vi "FlexRay_Demo.vi"(11 "Receiver":string="FlexRay_Demo") -> ()   [LabVIEW 2014]
uses:
  <vilib>/Utility/miscctls.llb/LVPointTypeDef.ctl
  TSMaster_API/FlexRay_Function/Typedef/FlexRay_Data.ctl
  TSMaster_API/FlexRay_Function/Typedef/TLibFLexRay.ctl
  TSMaster_API/FlexRay_Function/Typedef/FlexRay_Config.ctl
  TSMaster_API/DataBase/Typedef/FlexRay/TFlexRaySignal.ctl
  TSMaster_API/DataBase/Typedef/LIN/TLINSignal.ctl
  TSMaster_API/DataBase/Typedef/CAN/TCANSignal.ctl
  TSMaster_API/DataBase/Typedef/TDBSignalProperties.ctl
  TSMaster_API/DataBase/Typedef/TDBFrameProperties.ctl
  TSMaster_API/DataBase/Typedef/TDBECUProperties.ctl
  TSMaster_API/DataBase/Typedef/TDBProperties.ctl
  <vilib>/regexp/Match Regular Expression.xnode
  TSMaster_API/DataBase/Typedef/DataBase_array.ctl
  TSMaster_API/DataBase/Typedef/DataBase_array_index.ctl
panel:
  out "DataBase_array":T1
  in  "CH_Mapping":bool
  in  "TS_Mapping":bool
  in  "Diagram shown":bool
  out "FlexRay_Data":T9={"Communication message"={"Sender"="", "receiver"="", "message"="", "data"=variant}, "error in"={"status"=FALSE, "code"=0, "source"=""}, "Data"={"FR_Frame_Buffer"=[], "Config"={"DLL_PATH"=path "", "Project_PATH"=path "", "BLF_Log_PATH"=path "", "Read message type"=1, "Channel"=0, "REC_Channel"=0, "ChannelMask"=0, "ActualPayloadLength"=0, "CycleNumber"=0, "SlotId"=0, "Send_Array"=[1, 2, 3, 4, 5, 6, 7, 8, 9, 10, 11]}, "AsynCall?"=FALSE, "XML_Data"={"XML Path"=path "", "XML loading channel"=0}, "DataBase_array"=refnum}} {"Data"."XML_Data"."XML loading channel" items=["CHN1", "CHN2", "CHN3", "CHN4", "CHN5", "CHN6", "CHN7", "CHN8", "CHN9", "CHN10", "CHN11", "CHN12", "CHN13", "CHN14", "CHN15", "CHN16", "CHN17", "CHN18", "CHN19", "CHN20", "CHN21", "CHN22", "CHN23", "CHN24", "CHN25", "CHN26", "CHN27", "CHN28", "CHN29", "CHN30", "CHN31", "CHN32"]; "Data"."Config"."Send_Array" format="%.0x"; "Data"."Config"."ChannelMask" items=["reserved", "A", "B", "AB"]; "Data"."Config"."REC_Channel" items=["CHN1", "CHN2", "CHN3", "CHN4", "CHN5", "CHN6", "CHN7", "CHN8", "CHN9", "CHN10", "CHN11", "CHN12", "CHN13", "CHN14", "CHN15", "CHN16", "CHN17", "CHN18", "CHN19", "CHN20", "CHN21", "CHN22", "CHN23", "CHN24", "CHN25", "CHN26", "CHN27", "CHN28", "CHN29", "CHN30", "CHN31", "CHN32"]; "Data"."Config"."Channel" items=["CHN1", "CHN2", "CHN3", "CHN4", "CHN5", "CHN6", "CHN7", "CHN8", "CHN9", "CHN10", "CHN11", "CHN12", "CHN13", "CHN14", "CHN15", "CHN16", "CHN17", "CHN18", "CHN19", "CHN20", "CHN21", "CHN22", "CHN23", "CHN24", "CHN25", "CHN26", "CHN27", "CHN28", "CHN29", "CHN30", "CHN31", "CHN32"]; "Data"."Config"."Read message type" items=["Only read received messages", "Receive&send messages"]}
  in  "Stop Log":bool
  in  "Start Log":bool
  in  "Config":bool
  in  "Connect":bool
  in  "Disconnect":bool
  out "Connect ?":bool
  in  "Tab Control":enum32{"Setting", "FlexRay", "XML_load"}(tab)
  in  "BLF_Log_PATH":path
  in  "Project_PATH":path
  in  "DLL_PATH":path
  in  "Import":bool
  in  "Export":bool
  in  "Signals":string[][](array[string])
  in  "Messages":string(combo)
  in  "Fold Data":bool
  in  "Transmit":bool
  in  "Send_Array":u8[](array[numeric])=[1, 2, 3, 4, 5, 6, 7, 8, 9, 10, 11] format="%.0x"
  in  "SlotId":u16
  in  "CycleNumber":u8 caption="Base+Rep"
  in  "ActualPayloadLength":u8 caption="Length"
  in  "DIS_REC":bool
  in  "Clear":bool
  in  "Pause":bool
  in  "REC_Channel":i32(ring) items=["CHN1", "CHN2", "CHN3", "CHN4", "CHN5", "CHN6", "CHN7", "CHN8", "CHN9", "CHN10", "CHN11", "CHN12", "CHN13", "CHN14", "CHN15", "CHN16", "CHN17", "CHN18", "CHN19", "CHN20", "CHN21", "CHN22", "CHN23", "CHN24", "CHN25", "CHN26", "CHN27", "CHN28", "CHN29", "CHN30", "CHN31", "CHN32"]
  in  "Channel":i32(ring) caption="REC_Channel" items=["CHN1", "CHN2", "CHN3", "CHN4", "CHN5", "CHN6", "CHN7", "CHN8", "CHN9", "CHN10", "CHN11", "CHN12", "CHN13", "CHN14", "CHN15", "CHN16", "CHN17", "CHN18", "CHN19", "CHN20", "CHN21", "CHN22", "CHN23", "CHN24", "CHN25", "CHN26", "CHN27", "CHN28", "CHN29", "CHN30", "CHN31", "CHN32"]
  out "Receive Status":bool
  in  "Read message type":u16(ring)=1 items=["Only read received messages", "Receive&send messages"]
  in  "Receive_Data":i32(listbox)=-1 caption="Data"
  in  "ChannelMask":u16(ring) items=["reserved", "A", "B", "AB"]
  out "Laod XML Successful?":bool caption="Laod BDC Successful?"
  in  "Unload":bool
  in  "Load_XML":bool
  in  "XML loading channel":i32(ring) items=["CHN1", "CHN2", "CHN3", "CHN4", "CHN5", "CHN6", "CHN7", "CHN8", "CHN9", "CHN10", "CHN11", "CHN12", "CHN13", "CHN14", "CHN15", "CHN16", "CHN17", "CHN18", "CHN19", "CHN20", "CHN21", "CHN22", "CHN23", "CHN24", "CHN25", "CHN26", "CHN27", "CHN28", "CHN29", "CHN30", "CHN31", "CHN32"]
  in  "XML Path":path
  in  "XML Tab":enum32{"Message", "Signal"}(tab) caption="Tab Control 2"
  in  "Message Table":string[][](table)=[["Name", ""], ["ChannelMask", ""], ["BaseCycle", ""], ["CycleRepetition", ""], ["SlotId", ""], ["DLC", ""], ["", ""], ["", ""]]
  in  "Signal Table":string[][](table)
  in  "Tree control":string(tree)
  in  "Creat error":bool
  in  "log":i32(listbox)
  in  "Quit":bool
  # "FlexRay Demo"
  # "Please click the 'Config' button first,Don't click \"Connect\""
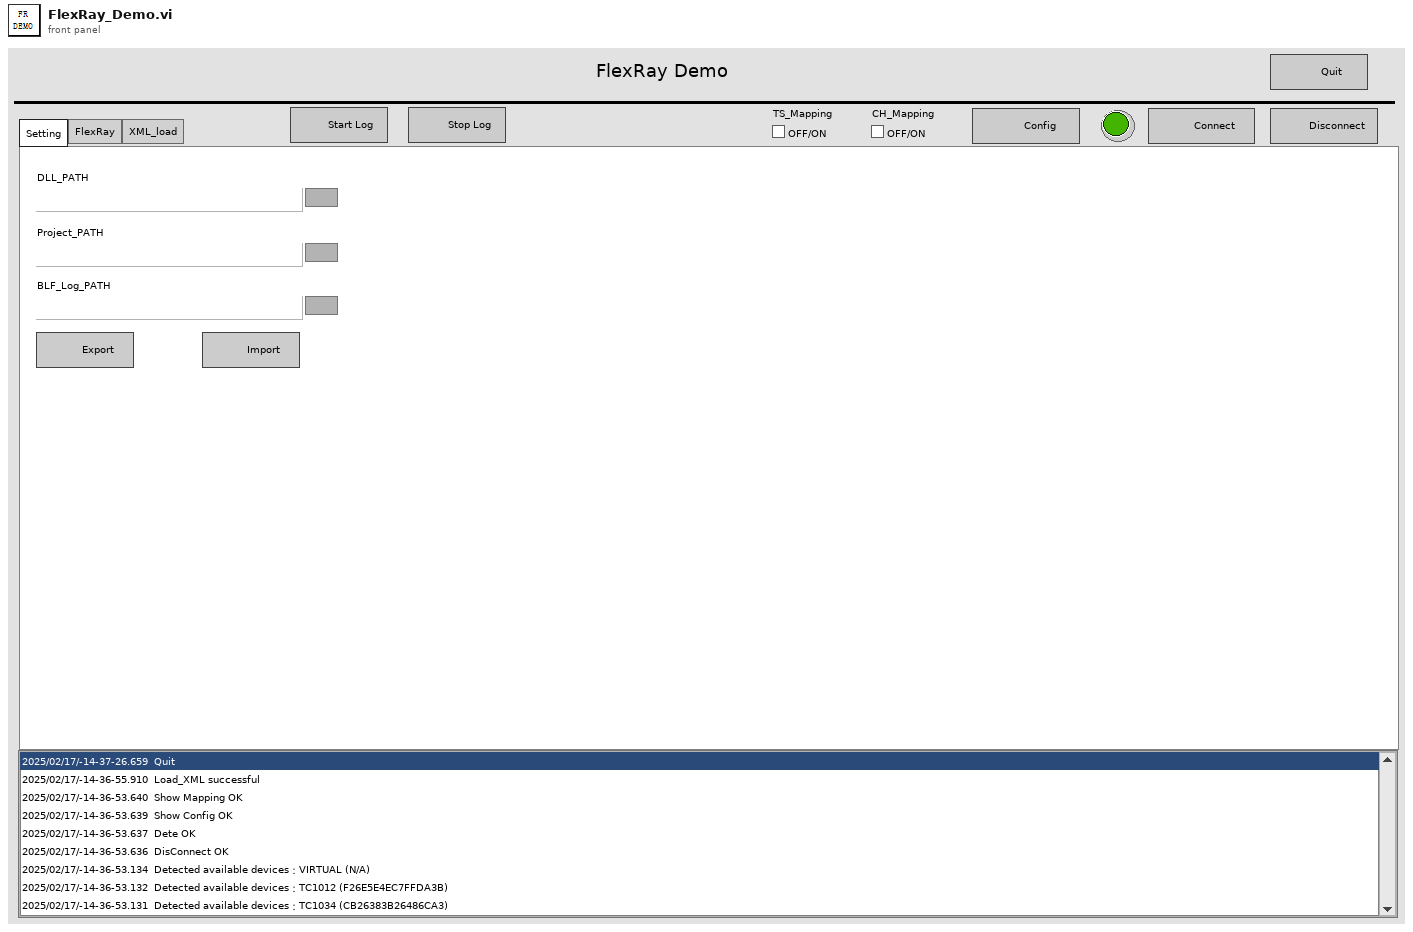
[diagram p1: front panel]
types:
  T1 = typedef "DataBase_array.ctl" = cluster{"db_properties":T2, "ECU_array":cluster{"TDBECUProperties":T3, "TX_Frame_array":cluster{"Frame_Properties":T4, "signal_array":T5[]}[], "RX_Frame_array":cluster{"Frame_Properties":T4, "signal_array":T5[]}[]}[]}[]
  T2 = typedef "TDBProperties.ctl" = cluster{"FDBIndex":i32, "FSignalCount":i32, "FFrameCount":i32, "FECUCount":i32, "FSupportedChannelMask":u64, "FName":cluster{"数值":u64, "数值 2":u64, "数值 3":u64, "数值 4":u64, "数值 5":u64, "数值 6":u64, "数值 7":u64, "数值 8":u64, "数值 9":u64, "数值 10":u64, "数值 11":u64, "数值 12":u64, "数值 13":u64, "数值 14":u64, "数值 15":u64, "数值 16":u64, "数值 17":u64, "数值 18":u64, "数值 19":u64, "数值 20":u64, "数值 21":u64, "数值 22":u64, "数值 23":u64, "数值 24":u64, "数值 25":u64, "数值 26":u64, "数值 27":u64, "数值 28":u64, "数值 29":u64, "数值 30":u64, "数值 31":u64, "数值 32":u64, "数值 33":u64, "数值 34":u64, "数值 35":u64, "数值 36":u64, "数值 37":u64, "数值 38":u64, "数值 39":u64, "数值 40":u64, "数值 41":u64, "数值 42":u64, "数值 43":u64, "数值 44":u64, "数值 45":u64, "数值 46":u64, "数值 47":u64, "数值 48":u64, "数值 49":u64, "数值 50":u64, "数值 51":u64, "数值 52":u64, "数值 53":u64, "数值 54":u64, "数值 55":u64, "数值 56":u64, "数值 57":u64, "数值 58":u64, "数值 59":u64, "数值 60":u64, "数值 61":u64, "数值 62":u64, "数值 63":u64, "数值 64":u64}, "FComment":cluster{"数值":u64, "数值 2":u64, "数值 3":u64, "数值 4":u64, "数值 5":u64, "数值 6":u64, "数值 7":u64, "数值 8":u64, "数值 9":u64, "数值 10":u64, "数值 11":u64, "数值 12":u64, "数值 13":u64, "数值 14":u64, "数值 15":u64, "数值 16":u64, "数值 17":u64, "数值 18":u64, "数值 19":u64, "数值 20":u64, "数值 21":u64, "数值 22":u64, "数值 23":u64, "数值 24":u64, "数值 25":u64, "数值 26":u64, "数值 27":u64, "数值 28":u64, "数值 29":u64, "数值 30":u64, "数值 31":u64, "数值 32":u64, "数值 33":u64, "数值 34":u64, "数值 35":u64, "数值 36":u64, "数值 37":u64, "数值 38":u64, "数值 39":u64, "数值 40":u64, "数值 41":u64, "数值 42":u64, "数值 43":u64, "数值 44":u64, "数值 45":u64, "数值 46":u64, "数值 47":u64, "数值 48":u64, "数值 49":u64, "数值 50":u64, "数值 51":u64, "数值 52":u64, "数值 53":u64, "数值 54":u64, "数值 55":u64, "数值 56":u64, "数值 57":u64, "数值 58":u64, "数值 59":u64, "数值 60":u64, "数值 61":u64, "数值 62":u64, "数值 63":u64, "数值 64":u64}, "FFlags":u32, "FDBId":u32}
  T3 = typedef "TDBECUProperties.ctl" = cluster{"FDBIndex":i32, "FECUIndex":i32, "FTxFrameCount":i32, "FRxFrameCount":i32, "FName":cluster{"数值":u64, "数值 2":u64, "数值 3":u64, "数值 4":u64, "数值 5":u64, "数值 6":u64, "数值 7":u64, "数值 8":u64, "数值 9":u64, "数值 10":u64, "数值 11":u64, "数值 12":u64, "数值 13":u64, "数值 14":u64, "数值 15":u64, "数值 16":u64, "数值 17":u64, "数值 18":u64, "数值 19":u64, "数值 20":u64, "数值 21":u64, "数值 22":u64, "数值 23":u64, "数值 24":u64, "数值 25":u64, "数值 26":u64, "数值 27":u64, "数值 28":u64, "数值 29":u64, "数值 30":u64, "数值 31":u64, "数值 32":u64, "数值 33":u64, "数值 34":u64, "数值 35":u64, "数值 36":u64, "数值 37":u64, "数值 38":u64, "数值 39":u64, "数值 40":u64, "数值 41":u64, "数值 42":u64, "数值 43":u64, "数值 44":u64, "数值 45":u64, "数值 46":u64, "数值 47":u64, "数值 48":u64, "数值 49":u64, "数值 50":u64, "数值 51":u64, "数值 52":u64, "数值 53":u64, "数值 54":u64, "数值 55":u64, "数值 56":u64, "数值 57":u64, "数值 58":u64, "数值 59":u64, "数值 60":u64, "数值 61":u64, "数值 62":u64, "数值 63":u64, "数值 64":u64}, "FComment":cluster{"数值":u64, "数值 2":u64, "数值 3":u64, "数值 4":u64, "数值 5":u64, "数值 6":u64, "数值 7":u64, "数值 8":u64, "数值 9":u64, "数值 10":u64, "数值 11":u64, "数值 12":u64, "数值 13":u64, "数值 14":u64, "数值 15":u64, "数值 16":u64, "数值 17":u64, "数值 18":u64, "数值 19":u64, "数值 20":u64, "数值 21":u64, "数值 22":u64, "数值 23":u64, "数值 24":u64, "数值 25":u64, "数值 26":u64, "数值 27":u64, "数值 28":u64, "数值 29":u64, "数值 30":u64, "数值 31":u64, "数值 32":u64, "数值 33":u64, "数值 34":u64, "数值 35":u64, "数值 36":u64, "数值 37":u64, "数值 38":u64, "数值 39":u64, "数值 40":u64, "数值 41":u64, "数值 42":u64, "数值 43":u64, "数值 44":u64, "数值 45":u64, "数值 46":u64, "数值 47":u64, "数值 48":u64, "数值 49":u64, "数值 50":u64, "数值 51":u64, "数值 52":u64, "数值 53":u64, "数值 54":u64, "数值 55":u64, "数值 56":u64, "数值 57":u64, "数值 58":u64, "数值 59":u64, "数值 60":u64, "数值 61":u64, "数值 62":u64, "数值 63":u64, "数值 64":u64}}
  T4 = typedef "TDBFrameProperties.ctl" = cluster{"FDBIndex":i32, "FECUIndex":i32, "FFrameIndex":i32, "FIsTx":u8, "FReserved1":u8, "FCycleTimeMs":u16, "TSignalType":i32, "FCANIsDataFrame":u8, "FCANIsStdFrame":u8, "FCANIsEdl":u8, "FCANIsBrs":u8, "FCANIdentifier":i32, "FCANDLC":i32, "FCANDataBytes":i32, "FLINIdentifier":i32, "FLINDLC":i32, "FFRChannelMask":u8, "FFRBaseCycle":u8, "FFRCycleRepetition":u8, "FFRIsStartupFrame":u8, "FFRSlotId":u16, "FFRDLC":u16, "FFRCycleMask":u64, "FSignalCount":i32, "FName":cluster{"数值":u64, "数值 2":u64, "数值 3":u64, "数值 4":u64, "数值 5":u64, "数值 6":u64, "数值 7":u64, "数值 8":u64, "数值 9":u64, "数值 10":u64, "数值 11":u64, "数值 12":u64, "数值 13":u64, "数值 14":u64, "数值 15":u64, "数值 16":u64, "数值 17":u64, "数值 18":u64, "数值 19":u64, "数值 20":u64, "数值 21":u64, "数值 22":u64, "数值 23":u64, "数值 24":u64, "数值 25":u64, "数值 26":u64, "数值 27":u64, "数值 28":u64, "数值 29":u64, "数值 30":u64, "数值 31":u64, "数值 32":u64, "数值 33":u64, "数值 34":u64, "数值 35":u64, "数值 36":u64, "数值 37":u64, "数值 38":u64, "数值 39":u64, "数值 40":u64, "数值 41":u64, "数值 42":u64, "数值 43":u64, "数值 44":u64, "数值 45":u64, "数值 46":u64, "数值 47":u64, "数值 48":u64, "数值 49":u64, "数值 50":u64, "数值 51":u64, "数值 52":u64, "数值 53":u64, "数值 54":u64, "数值 55":u64, "数值 56":u64, "数值 57":u64, "数值 58":u64, "数值 59":u64, "数值 60":u64, "数值 61":u64, "数值 62":u64, "数值 63":u64, "数值 64":u64}, "FComment":cluster{"数值":u64, "数值 2":u64, "数值 3":u64, "数值 4":u64, "数值 5":u64, "数值 6":u64, "数值 7":u64, "数值 8":u64, "数值 9":u64, "数值 10":u64, "数值 11":u64, "数值 12":u64, "数值 13":u64, "数值 14":u64, "数值 15":u64, "数值 16":u64, "数值 17":u64, "数值 18":u64, "数值 19":u64, "数值 20":u64, "数值 21":u64, "数值 22":u64, "数值 23":u64, "数值 24":u64, "数值 25":u64, "数值 26":u64, "数值 27":u64, "数值 28":u64, "数值 29":u64, "数值 30":u64, "数值 31":u64, "数值 32":u64, "数值 33":u64, "数值 34":u64, "数值 35":u64, "数值 36":u64, "数值 37":u64, "数值 38":u64, "数值 39":u64, "数值 40":u64, "数值 41":u64, "数值 42":u64, "数值 43":u64, "数值 44":u64, "数值 45":u64, "数值 46":u64, "数值 47":u64, "数值 48":u64, "数值 49":u64, "数值 50":u64, "数值 51":u64, "数值 52":u64, "数值 53":u64, "数值 54":u64, "数值 55":u64, "数值 56":u64, "数值 57":u64, "数值 58":u64, "数值 59":u64, "数值 60":u64, "数值 61":u64, "数值 62":u64, "数值 63":u64, "数值 64":u64}}
  T5 = typedef "TDBSignalProperties.ctl" = cluster{"FDBIndex":i32, "FECUIndex":i32, "FFrameIndex":i32, "FSignalIndex":i32, "FIsTx":u8, "FReserved1":u8, "FReserved2":u8, "FReserved3":u8, "TSignalType":i32, "TCANSignal":T6, "TLINSignal":T7, "TFlexRaySignal":T8, "FParentFrameId":i32, "FInitValue":dbl, "FName":cluster{"数值":u64, "数值 2":u64, "数值 3":u64, "数值 4":u64, "数值 5":u64, "数值 6":u64, "数值 7":u64, "数值 8":u64, "数值 9":u64, "数值 10":u64, "数值 11":u64, "数值 12":u64, "数值 13":u64, "数值 14":u64, "数值 15":u64, "数值 16":u64, "数值 17":u64, "数值 18":u64, "数值 19":u64, "数值 20":u64, "数值 21":u64, "数值 22":u64, "数值 23":u64, "数值 24":u64, "数值 25":u64, "数值 26":u64, "数值 27":u64, "数值 28":u64, "数值 29":u64, "数值 30":u64, "数值 31":u64, "数值 32":u64, "数值 33":u64, "数值 34":u64, "数值 35":u64, "数值 36":u64, "数值 37":u64, "数值 38":u64, "数值 39":u64, "数值 40":u64, "数值 41":u64, "数值 42":u64, "数值 43":u64, "数值 44":u64, "数值 45":u64, "数值 46":u64, "数值 47":u64, "数值 48":u64, "数值 49":u64, "数值 50":u64, "数值 51":u64, "数值 52":u64, "数值 53":u64, "数值 54":u64, "数值 55":u64, "数值 56":u64, "数值 57":u64, "数值 58":u64, "数值 59":u64, "数值 60":u64, "数值 61":u64, "数值 62":u64, "数值 63":u64, "数值 64":u64}, "FComment":cluster{"数值":u64, "数值 2":u64, "数值 3":u64, "数值 4":u64, "数值 5":u64, "数值 6":u64, "数值 7":u64, "数值 8":u64, "数值 9":u64, "数值 10":u64, "数值 11":u64, "数值 12":u64, "数值 13":u64, "数值 14":u64, "数值 15":u64, "数值 16":u64, "数值 17":u64, "数值 18":u64, "数值 19":u64, "数值 20":u64, "数值 21":u64, "数值 22":u64, "数值 23":u64, "数值 24":u64, "数值 25":u64, "数值 26":u64, "数值 27":u64, "数值 28":u64, "数值 29":u64, "数值 30":u64, "数值 31":u64, "数值 32":u64, "数值 33":u64, "数值 34":u64, "数值 35":u64, "数值 36":u64, "数值 37":u64, "数值 38":u64, "数值 39":u64, "数值 40":u64, "数值 41":u64, "数值 42":u64, "数值 43":u64, "数值 44":u64, "数值 45":u64, "数值 46":u64, "数值 47":u64, "数值 48":u64, "数值 49":u64, "数值 50":u64, "数值 51":u64, "数值 52":u64, "数值 53":u64, "数值 54":u64, "数值 55":u64, "数值 56":u64, "数值 57":u64, "数值 58":u64, "数值 59":u64, "数值 60":u64, "数值 61":u64, "数值 62":u64, "数值 63":u64, "数值 64":u64}}
  T6 = typedef "TCANSignal.ctl" = cluster{"FCANSgnType":u8, "FIsIntel":u8, "FStartBit":i32, "FLength":i32, "FFactor":dbl, "FOffset":dbl}
  T7 = typedef "TLINSignal.ctl" = cluster{"FLINSgnType":u8, "FIsIntel":u8, "FStartBit":i32, "FLength":i32, "FFactor":dbl, "FOffset":dbl}
  T8 = typedef "TFlexRaySignal.ctl" = cluster{"FFRSgnType":u8, "FCompuMethod":u8, "FReserved":u8, "FIsIntel":u8, "FStartBit":i32, "FUpdateBit":i32, "FLength":i32, "FFactor":dbl, "FOffset":dbl, "FActualStartBit":i32, "FActualUpdateBit":i32}
  T9 = typedef "FlexRay_Data.ctl" = cluster{"Communication message":cluster{"Sender":string, "receiver":string, "message":string, "data":variant}, "error in":errorcluster, "Data":cluster{"FR_Frame_Buffer":T10[], "Config":T11, "AsynCall?":bool, "XML_Data":cluster{"XML Path":path, "XML loading channel":i32}, "DataBase_array":T12}}
  T10 = typedef "TLibFLexRay.ctl" = cluster{"FIdxChn":u8, "FChannelMask":u8, "FDir":u8, "FPayloadLength":u8, "FActualPayloadLength":u8, "FCycleNumber":u8, "FCCType":u8, "FFrameType":u8, "FHeaderCRCA":u16, "FHeaderCRCB":u16, "FFrameStateInfo":u16, "FSlotId":u16, "FFrameFlags":u32, "FFrameCRC":u32, "FReserved1":u64, "FReserved2":u64, "FTimeUs":u64, "FData":cluster{"数值":u8, "数值 9":u8, "数值 17":u8, "数值 25":u8, "数值 33":u8, "数值 41":u8, "数值 49":u8, "数值 57":u8, "数值 65":u8, "数值 73":u8, "数值 81":u8, "数值 89":u8, "数值 97":u8, "数值 105":u8, "数值 98":u8, "数值 99":u8, "数值 2":u8, "数值 10":u8, "数值 18":u8, "数值 26":u8, "数值 34":u8, "数值 42":u8, "数值 50":u8, "数值 58":u8, "数值 66":u8, "数值 74":u8, "数值 82":u8, "数值 90":u8, "数值 100":u8, "数值 106":u8, "数值 101":u8, "数值 102":u8, "数值 3":u8, "数值 11":u8, "数值 19":u8, "数值 27":u8, "数值 35":u8, "数值 43":u8, "数值 51":u8, "数值 59":u8, "数值 67":u8, "数值 75":u8, "数值 83":u8, "数值 91":u8, "数值 103":u8, "数值 107":u8, "数值 104":u8, "数值 108":u8, "数值 4":u8, "数值 12":u8, "数值 20":u8, "数值 28":u8, "数值 36":u8, "数值 44":u8, "数值 52":u8, "数值 60":u8, "数值 68":u8, "数值 76":u8, "数值 84":u8, "数值 92":u8, "数值 109":u8, "数值 110":u8, "数值 111":u8, "数值 112":u8, "数值 5":u8, "数值 13":u8, "数值 21":u8, "数值 29":u8, "数值 37":u8, "数值 45":u8, "数值 53":u8, "数值 61":u8, "数值 69":u8, "数值 77":u8, "数值 85":u8, "数值 93":u8, "数值 113":u8, "数值 114":u8, "数值 115":u8, "数值 116":u8, "数值 6":u8, "数值 14":u8, "数值 22":u8, "数值 30":u8, "数值 38":u8, "数值 46":u8, "数值 54":u8, "数值 62":u8, "数值 70":u8, "数值 78":u8, "数值 86":u8, "数值 94":u8, "数值 117":u8, "数值 118":u8, "数值 119":u8, "数值 120":u8, "数值 7":u8, "数值 15":u8, "数值 23":u8, "数值 31":u8, "数值 39":u8, "数值 47":u8, "数值 55":u8, "数值 63":u8, "数值 71":u8, "数值 79":u8, "数值 87":u8, "数值 95":u8, "数值 121":u8, "数值 122":u8, "数值 123":u8, "数值 124":u8, "数值 8":u8, "数值 16":u8, "数值 24":u8, "数值 32":u8, "数值 40":u8, "数值 48":u8, "数值 56":u8, "数值 64":u8, "数值 72":u8, "数值 80":u8, "数值 88":u8, "数值 96":u8, "数值 125":u8, "数值 126":u8, "数值 127":u8, "数值 128":u8, "数值 129":u8, "数值 130":u8, "数值 131":u8, "数值 132":u8, "数值 133":u8, "数值 134":u8, "数值 135":u8, "数值 136":u8, "数值 137":u8, "数值 138":u8, "数值 139":u8, "数值 140":u8, "数值 141":u8, "数值 142":u8, "数值 143":u8, "数值 144":u8, "数值 145":u8, "数值 146":u8, "数值 147":u8, "数值 148":u8, "数值 149":u8, "数值 150":u8, "数值 151":u8, "数值 152":u8, "数值 153":u8, "数值 154":u8, "数值 155":u8, "数值 156":u8, "数值 157":u8, "数值 158":u8, "数值 159":u8, "数值 160":u8, "数值 161":u8, "数值 162":u8, "数值 163":u8, "数值 164":u8, "数值 165":u8, "数值 166":u8, "数值 167":u8, "数值 168":u8, "数值 169":u8, "数值 170":u8, "数值 171":u8, "数值 172":u8, "数值 173":u8, "数值 174":u8, "数值 175":u8, "数值 176":u8, "数值 177":u8, "数值 178":u8, "数值 179":u8, "数值 180":u8, "数值 181":u8, "数值 182":u8, "数值 183":u8, "数值 184":u8, "数值 185":u8, "数值 186":u8, "数值 187":u8, "数值 188":u8, "数值 189":u8, "数值 190":u8, "数值 191":u8, "数值 192":u8, "数值 193":u8, "数值 194":u8, "数值 195":u8, "数值 196":u8, "数值 197":u8, "数值 198":u8, "数值 199":u8, "数值 200":u8, "数值 201":u8, "数值 202":u8, "数值 203":u8, "数值 204":u8, "数值 205":u8, "数值 206":u8, "数值 207":u8, "数值 208":u8, "数值 209":u8, "数值 210":u8, "数值 211":u8, "数值 212":u8, "数值 213":u8, "数值 214":u8, "数值 215":u8, "数值 216":u8, "数值 217":u8, "数值 218":u8, "数值 219":u8, "数值 220":u8, "数值 221":u8, "数值 222":u8, "数值 223":u8, "数值 224":u8, "数值 225":u8, "数值 226":u8, "数值 227":u8, "数值 228":u8, "数值 229":u8, "数值 230":u8, "数值 231":u8, "数值 232":u8, "数值 233":u8, "数值 234":u8, "数值 235":u8, "数值 236":u8, "数值 237":u8, "数值 238":u8, "数值 239":u8, "数值 241":u8, "数值 242":u8, "数值 243":u8, "数值 244":u8, "数值 245":u8, "数值 246":u8, "数值 247":u8, "数值 248":u8, "数值 249":u8, "数值 250":u8, "数值 251":u8, "数值 252":u8, "数值 253":u8, "数值 254":u8, "数值 255":u8}}
  T11 = typedef "FlexRay_Config.ctl" = cluster{"DLL_PATH":path, "Project_PATH":path, "BLF_Log_PATH":path, "Read message type":u16, "Channel":i32, "REC_Channel":i32, "ChannelMask":u16, "ActualPayloadLength":u8, "CycleNumber":u8, "SlotId":u16, "Send_Array":u8[]}
  T12 = typedef "DataBase_array_index.ctl" = refnum<vi>
  T13 = typedef "LVPointTypeDef.ctl" = cluster{"Horizontal":i16, "Vertical":i16}
  T14 = enum8{"Enabled", "Disabled", "Disabled and Grayed Out"}
  T15 = cluster{"Sender":string, "receiver":string, "message":string, "data":variant}
  T16 = cluster{"FIdxChn":u8, "FChannelMask":u8, "FActualPayloadLength":u8, "FCycleNumber":u8, "FSlotId":u16, "Send_Array":u8[]}
  T17 = cluster{"Frame_Properties":T4, "signal_array":T5[]}
  T18 = cluster{"FR_Frame_Buffer":T10[], "Config":T11, "AsynCall?":bool, "XML_Data":cluster{"XML Path":path, "XML loading channel":i32}, "DataBase_array":T12}
  T19 = enum32{"invalid app kind", "Development System", "Run Time System", "Student Edition", "Embedded LabVIEW", "Evaluation", "Custom"}
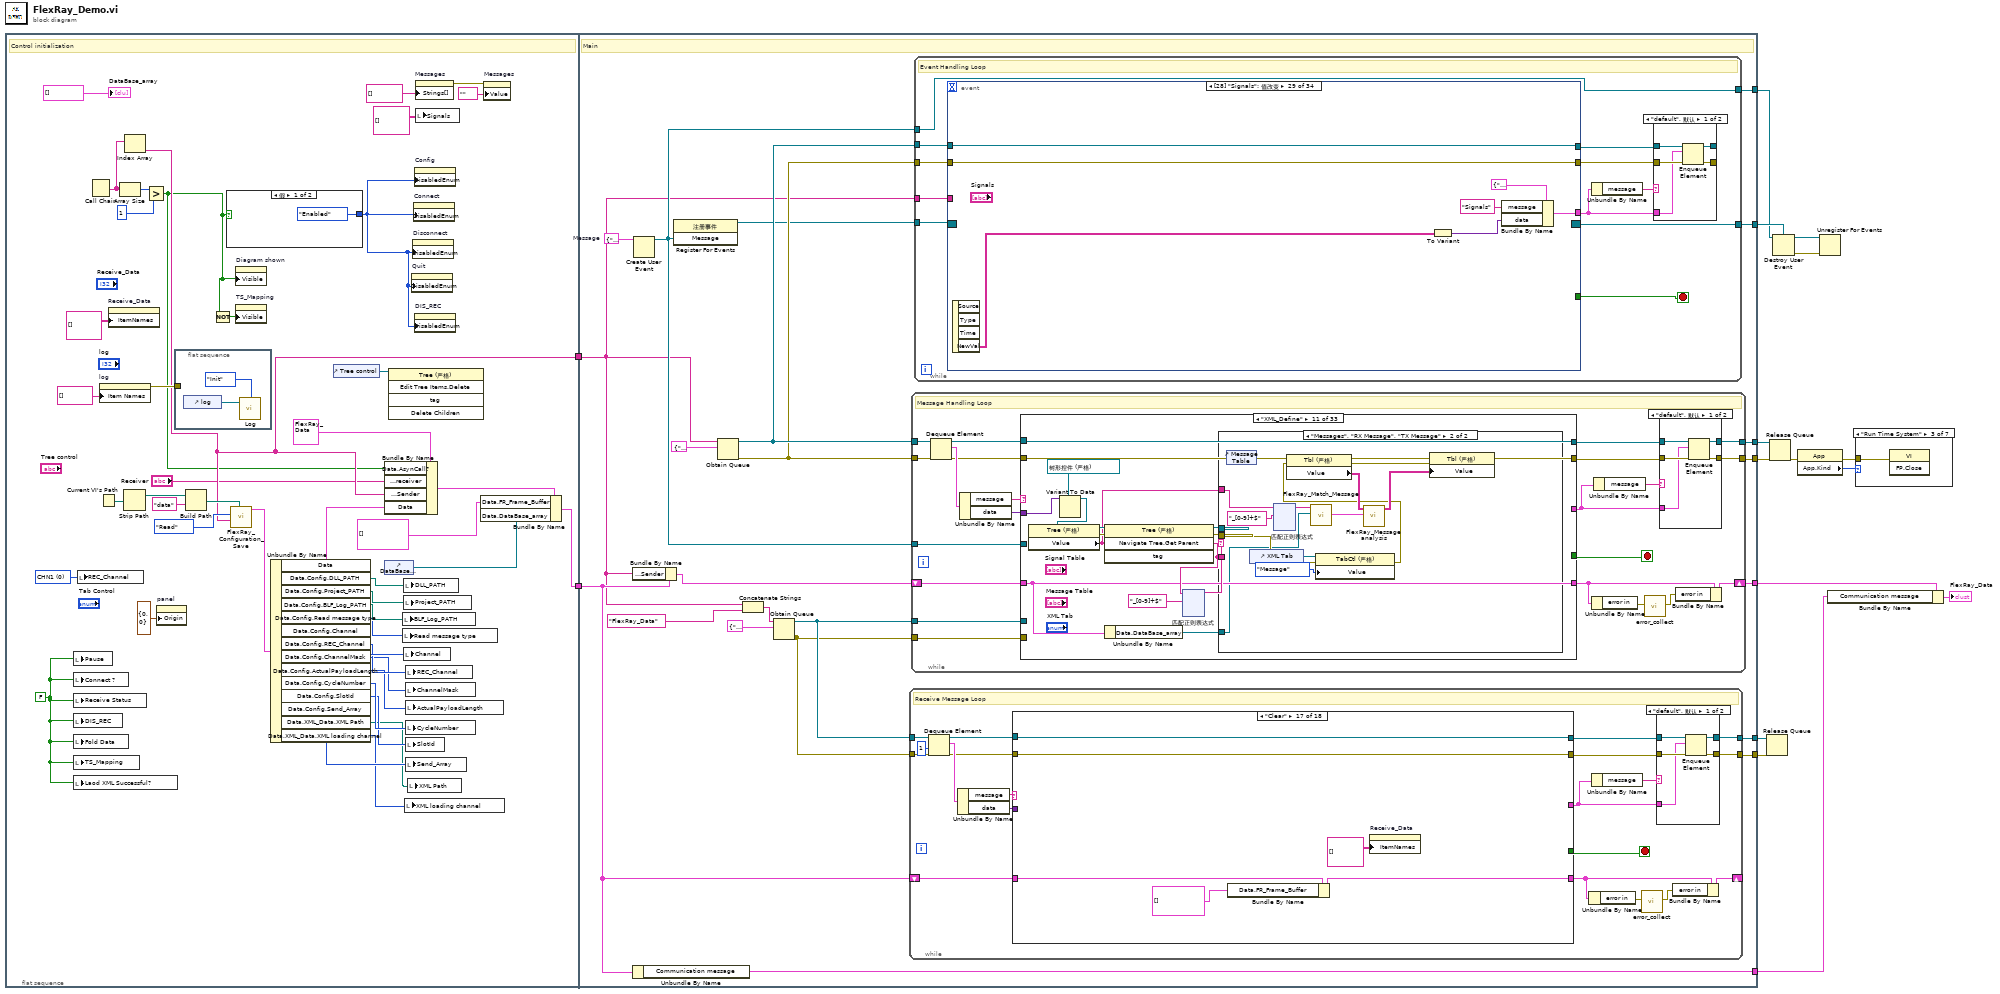
[diagram p0: block diagram]
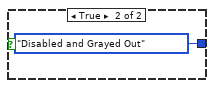
[diagram p2: hidden frame]
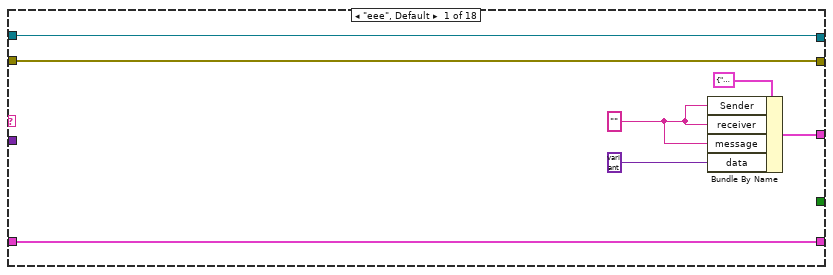
[diagram p4: hidden frame]
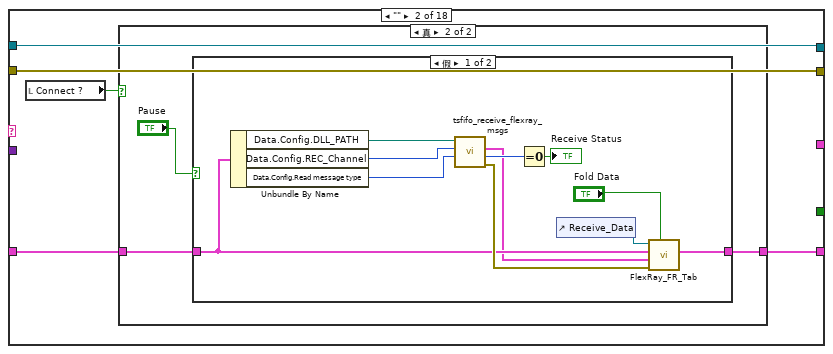
[diagram p5: hidden frame]
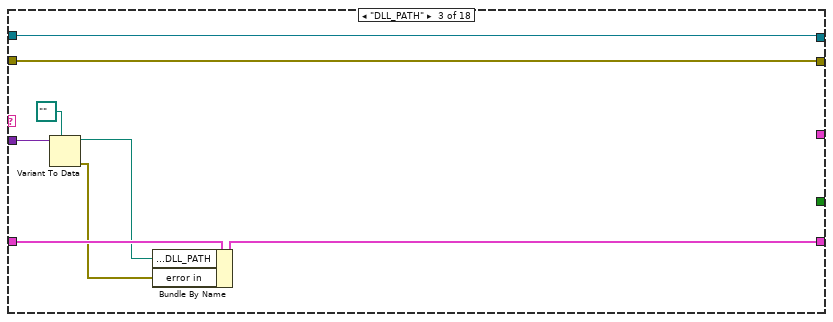
[diagram p8: hidden frame]
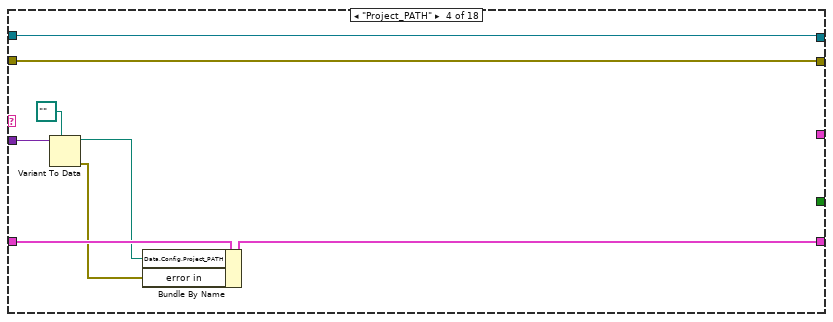
[diagram p9: hidden frame]
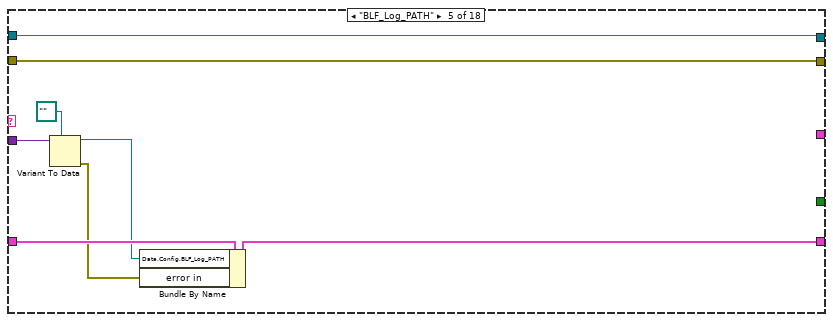
[diagram p10: hidden frame]
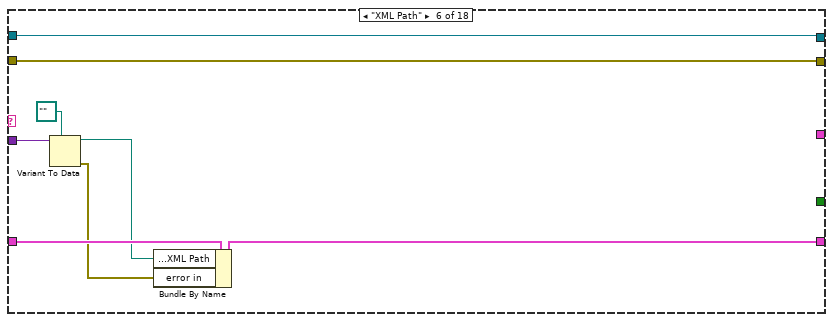
[diagram p11: hidden frame]
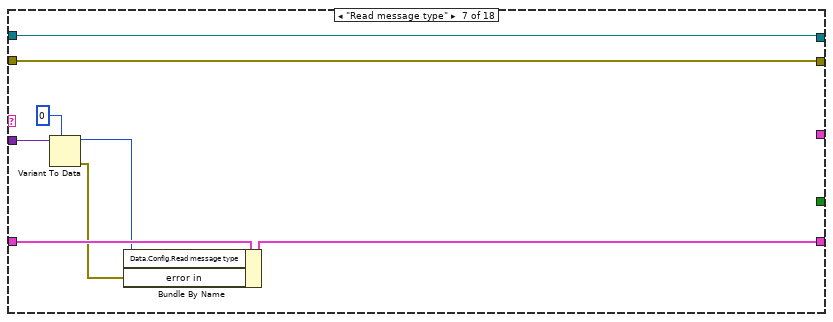
[diagram p12: hidden frame]
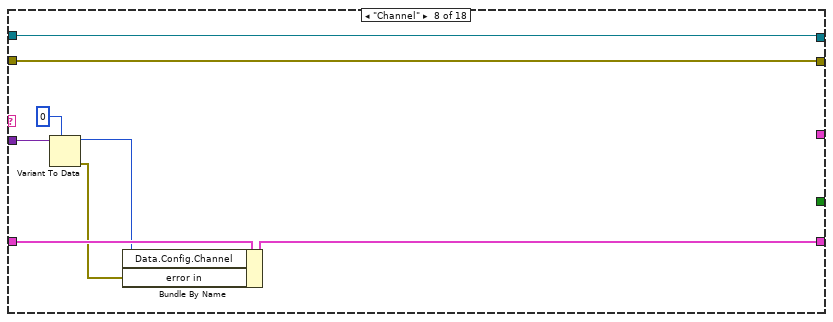
[diagram p13: hidden frame]
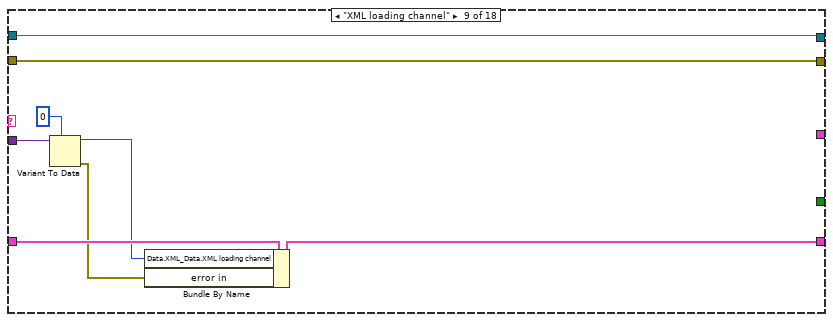
[diagram p14: hidden frame]
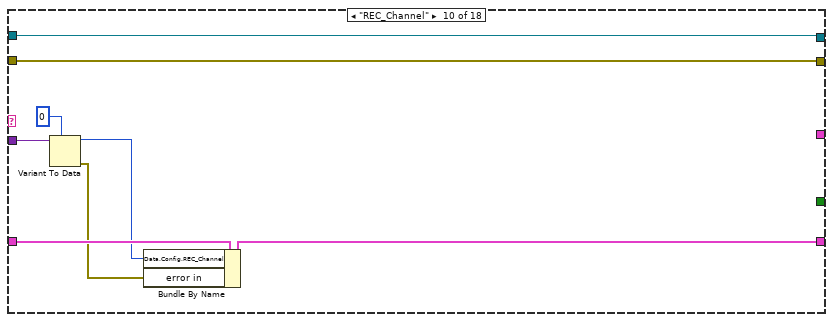
[diagram p15: hidden frame]
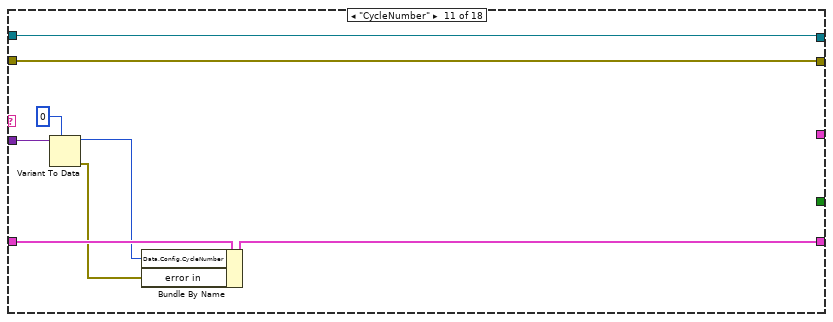
[diagram p16: hidden frame]
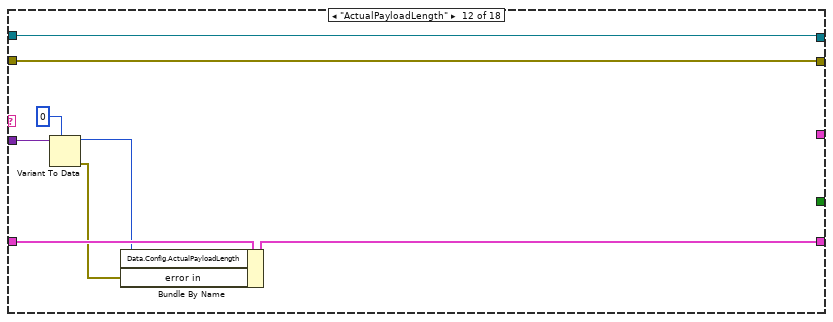
[diagram p17: hidden frame]
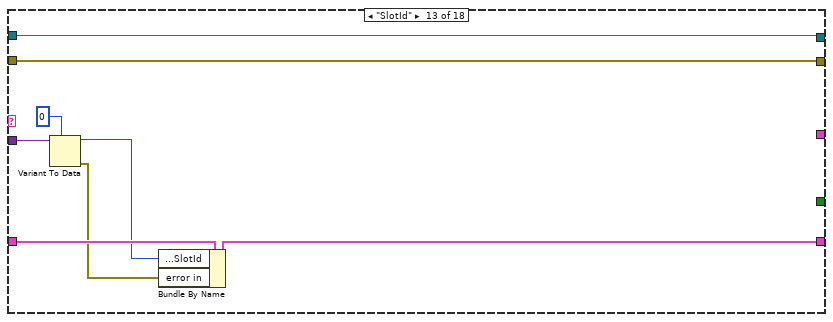
[diagram p18: hidden frame]
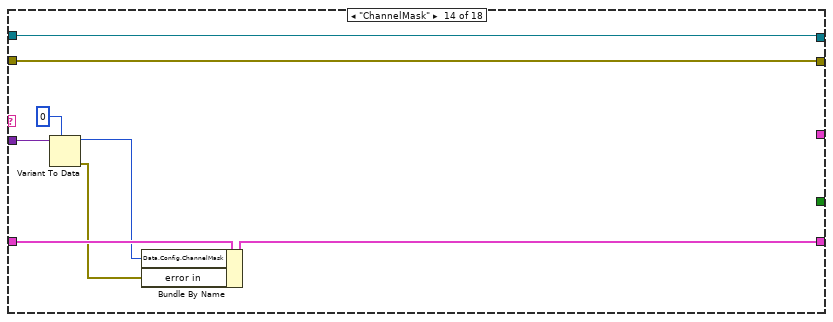
[diagram p19: hidden frame]
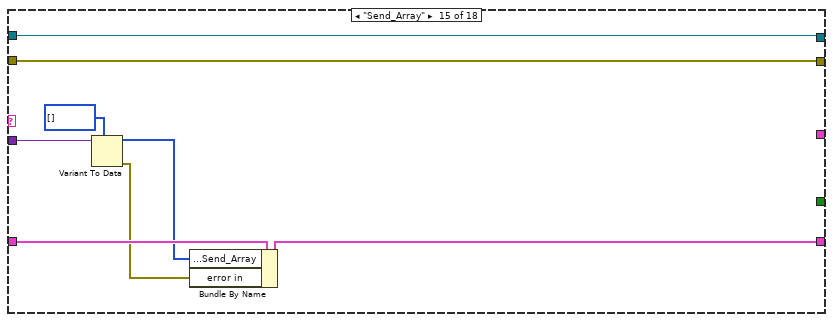
[diagram p20: hidden frame]
diagram:
  n1 = flat-sequence {
    tunnel: [w19] -> w3
    tunnel: [w33] -> w2
    tunnel: [w85] -> w15
    tunnel: [w84] -> w14
    tunnel: [w79] -> w10
    tunnel: [w77] -> w8
    tunnel: [w76] -> w7
    tunnel: [w70] -> w6
    tunnel: [w69] -> w5
    tunnel: w3 -> [w67]
    tunnel: w2 -> [w66]
    tunnel: [w68] -> w1
    frame #0 {
      w45 = 0 items=["CHN1", "CHN2", "CHN3", "CHN4", "CHN5", "CHN6", "CHN7", "CHN8", "CHN9", "CHN10", "CHN11", "CHN12", "CHN13", "CHN14", "CHN15", "CHN16", "CHN17", "CHN18", "CHN19", "CHN20", "CHN21", "CHN22", "CHN23", "CHN24", "CHN25", "CHN26", "CHN27", "CHN28", "CHN29", "CHN30", "CHN31", "CHN32"] ("REC_Channel")
      w28 = FALSE ("Connect ?")
      # "Control initialization"
      n2 = local write "Pause"(w28) -> ()
      n3 = local write "Connect ?"(w28) -> ()
      n4 = local write "Receive Status"(w28) -> ()
      n5 = local write "DIS_REC"(w28) -> ()
      n6 = local write "Fold Data"(w28) -> ()
      n7 = local write "TS_Mapping"(w28) -> ()
      n8 = local write "Laod XML Successful?"(w28) -> ()
      n9 = local write "REC_Channel"(w45) -> ()
      n10 = Call Chain() -> (call chain=w34:string[])
      n11 = Current VI's Path() -> (path=w56:path)
      n12 = property on="log" class="LstBox (严格)"("Item Names"=string[] [] ("项名")) -> (error out=w55:errorcluster)  [unwired: 2 in, 1 out]
      n13 = property on="Receive_Data" class="MCListbox (严格)"("ItemNames"=string[][] [] ("项名")) -> ()  [unwired: 2 in, 2 out]
      n14 = Array Size(array=w34) -> (size(s)=w36:i32)
      n15 = Strip Path(path=w56) -> (stripped path=w57:path)  [unwired: 1 out]
      n16 = Index Array(array=w34) -> (element=w33:string)  [unwired: 1 in]
      n17 = Greater?(x=w36, y=1) -> (0:w30:bool)
      n18 = property on="panel" class="Pane"("Origin"=T13 {"Horizontal"=0, "Vertical"=0} ("原点")) -> ()  [unwired: 2 in, 2 out]
      n19 = flat-sequence {
        tunnel: w55 -> [_]
        frame #0 {
          n20 = control-ref of="log"() -> (w63:refnum<vi>)
          n21 = call "Log.vi"("Method"=enum16{"Init", "Log"}."Init", "ListBox in"=w63) -> ()  [unwired: 2 in]
        }
      }
      n22 = Build Path(base path=w57, name or relative path="data") -> (appended path=w58:path)
      n23 = Not(x=w30) -> (.not. x?=w29:bool)
      n24 = case shown="假" w30 {
        tunnel: [T14."Enabled" ("禁用") T14."Disabled and Grayed Out" ("禁用")] -> w31
        frame False {
        }
        frame True {
        }
      }
      n25 = call "FlexRay_Configuration_Save.vi"("path"=w58, "Config Name"=w33, "Read/Write"=enum16{"Read", "Write"}."Read") -> ("FlexRay_Data"=w59:T9)  [unwired: 6 in, 2 out]
      n26 = property on="Diagram shown" class="Bool (严格)"("Visible"=w30) -> ()  [unwired: 2 in, 2 out]
      n27 = property on="TS_Mapping" class="Bool (严格)"("Visible"=w29) -> ()  [unwired: 2 in, 2 out]
      n28 = Unbundle By Name(w59) -> ("Data"=w60:T18, "Data.Config.DLL_PATH"=w49:path, "Data.Config.Project_PATH"=w48:path, "Data.Config.BLF_Log_PATH"=w47:path, "Data.Config.Read message type"=w46:u16, "Data.Config.Channel"=w44:i32, "Data.Config.REC_Channel"=w42:i32, "Data.Config.ChannelMask"=w41:u16, "Data.Config.ActualPayloadLength"=w40:u8, "Data.Config.CycleNumber"=w39:u8, "Data.Config.SlotId"=w38:u16, "Data.Config.Send_Array"=w37:u8[], "Data.XML_Data.XML Path"=w27:path, "Data.XML_Data.XML loading channel"=w26:i32)
      n29 = control-ref of="Tree control"() -> (w21:refnum<vi>)
      n30 = control-ref of="DataBase_array"() -> (w16:refnum<vi>)
      n31 = Bundle By Name(cluster=T9 {"Communication message"={"Sender"="", "receiver"="", "message"="", "data"=variant}, "error in"={"status"=FALSE, "code"=0, "source"=""}, "Data"={"FR_Frame_Buffer"=[], "Config"={"DLL_PATH"=path "", "Project_PATH"=path "", "BLF_Log_PATH"=path "", "Read message type"=1, "Channel"=0, "REC_Channel"=0, "ChannelMask"=0, "ActualPayloadLength"=0, "CycleNumber"=0, "SlotId"=0, "Send_Array"=[1, 2, 3, 4, 5, 6, 7, 8, 9, 10, 11]}, "AsynCall?"=FALSE, "XML_Data"={"XML Path"=path "", "XML loading channel"=0}, "DataBase_array"=refnum}} ("Data"), "Data.AsynCall?"=w30, "Communication message.receiver"="Receiver", "Communication message.Sender"=w33, "Data"=w60) -> (w50:T9)
      n32 = invoke class="Tree (严格)" method="Edit Tree Items.Delete"(reference=w21) -> ()  [unwired: 4 in, 5 out]
      n33 = local write "BLF_Log_PATH"(w47) -> ()
      n34 = local write "Read message type"(w46) -> ()
      n35 = local write "DLL_PATH"(w49) -> ()
      n36 = local write "Project_PATH"(w48) -> ()
      n37 = local write "Channel"(w44) -> ()
      n38 = local write "XML loading channel"(w26) -> ()
      n39 = local write "REC_Channel"(w42) -> ()
      n40 = local write "ChannelMask"(w41) -> ()
      n41 = local write "ActualPayloadLength"(w40) -> ()
      n42 = local write "CycleNumber"(w39) -> ()
      n43 = local write "SlotId"(w38) -> ()
      n44 = local write "Send_Array"(w37) -> ()
      n45 = local write "XML Path"(w27) -> ()
      n46 = property on="Quit" class="Bool"("DisabledEnum"=w31) -> ()  [unwired: 2 in, 2 out]
      n47 = property on="Disconnect" class="Bool"("DisabledEnum"=w31) -> ()  [unwired: 2 in, 2 out]
      n48 = property on="Connect" class="Bool"("DisabledEnum"=w31) -> ()  [unwired: 2 in, 2 out]
      n49 = property on="Config" class="Bool"("DisabledEnum"=w31) -> ()  [unwired: 2 in, 2 out]
      n50 = property on="DIS_REC" class="Bool (严格)"("DisabledEnum"=w31) -> ()  [unwired: 2 in, 2 out]
      n51 = property on="Messages" class="CmbBox"("Strings[]"=string[] [] ("字符串[]")) -> (error out=w22:errorcluster)  [unwired: 2 in, 1 out]
      n52 = local write "Signals"(string[][] [] ("Signals")) -> ()
      n53 = Bundle By Name(cluster=w50, "Data.FR_Frame_Buffer"=T10[] [], "Data.DataBase_array"=w16) -> (w19:T9)
      n54 = property on="Messages" class="CmbBox"(error in=w22, "Value"="" ("Messages")) -> ()  [unwired: 1 in, 2 out]
      "DataBase_array" <- T1 [] ("值")
    }
    frame #1 {
      w65 = T15 {"Sender"="", "receiver"="", "message"="", "data"=variant}  # Message
      # "Main"
      n55 = Bundle By Name(cluster=w67, "Communication message.Sender"=w66) -> (w81:T9)
      n56 = Unbundle By Name(w67) -> ("Communication message"=w68:T15)
      n57 = Create User Event(user event datatype=w65) -> (user event=w78:refnum<user-event>)  [unwired: 1 in, 1 out]
      n58 = register-events(w78) -> (reference out=w80:refnum<event-registration>)  [unwired: 2 in, 1 out]
      n59 = Obtain Queue(name (unnamed)=w66, element data type=T15 {"Sender"="", "receiver"="", "message"="", "data"=variant} ("Communication message")) -> (queue out=w86:refnum<queue>, error out=w82:errorcluster)  [unwired: 3 in, 1 out]
      n60 = Concatenate Strings(w66, "FlexRay_Data" ("字符串")) -> (w74:string)
      n61 = Obtain Queue(name (unnamed)=w74, element data type=T15 {"Sender"="", "receiver"="", "message"="", "data"=variant} ("Communication message")) -> (queue out=w72:refnum<queue>, error out=w71:errorcluster)  [unwired: 3 in, 1 out]
      n62 = while {
        tunnel: w72 -> [w106]
        tunnel: w71 -> [w105]
        tunnel: [w97] -> w70
        tunnel: [w96] -> w69
        shift-right: [w89] -> _
        shift-left: w67 -> [w92]
        stop <- w95 stop-if-true
        # "Receive Message Loop"
        n63 = Dequeue Element(queue=w106, timeout in ms (-1)=1, error in (no error)=w105) -> (queue out=w102:refnum<queue>, element=w104:T15, error out=w101:errorcluster)  [unwired: 1 out]
        n64 = Unbundle By Name(w104) -> ("message"=w103:string, "data"=w98:variant)
        n65 = case shown="\"Clear\"" w103 {
          tunnel: [w120 w125 w149 w157 w165 w173 w181 w189 w197 w205 w213 w221 w229 w237 w245 w253 w259 w262] -> w100
          tunnel: w102 -> [w120 w125 w149 w157 w165 w173 w181 w189 w197 w205 w213 w221 w229 w237 w245 w253 w259 w262]
          tunnel: w101 -> [w119 w124 w148 w156 w164 w172 w180 w188 w196 w204 w212 w220 w228 w236 w244 w252 w258 w261]
          tunnel: [w119 w124 w148 w156 w164 w172 w180 w188 w196 w204 w212 w220 w228 w236 w244 w252 w258 w261] -> w99
          tunnel: w98 -> [_ _ w146 w154 w162 w170 w178 w186 w194 w202 w210 w218 w226 w234 w242 w248 _ _]
          tunnel: [_ _ _ _ _ _ _ _ _ _ _ _ _ _ _ _ _ TRUE] -> w95
          tunnel: [w117 _ _ _ _ _ _ _ _ _ _ _ _ _ _ _ _ _] -> w94
          tunnel: [w114 w121 w144 w152 w160 w168 w177 w185 w193 w201 w209 w217 w225 w233 w241 w246 w256 w260] -> w91
          tunnel: w92 -> [w114 w123 w147 w155 w163 w171 w179 w187 w195 w203 w211 w219 w227 w235 w243 w247 w257 w260]
          frame "eee", Default {
            w115 = ""
            n66 = Bundle By Name(cluster=T15 {"Sender"="", "receiver"="", "message"="", "data"=variant} ("Communication message"), "Sender"=w115, "receiver"=w115, "message"=w115, "data"=variant) -> (w117:T15)
          }
          frame "" {
            n67 = local read "Connect ?"() -> (w122:bool)
            n68 = case shown="真" w122 {
              tunnel: w123 -> [w126 w129]
              tunnel: [w126 w128] -> w121
              frame False {
              }
              frame True {
                n69 = case shown="假" "Pause" {
                  tunnel: w129 -> [w135 w141]
                  tunnel: [w134 w141] -> w128
                  frame False {
                    n70 = Unbundle By Name(w135) -> ("Data.Config.DLL_PATH"=w131:path, "Data.Config.REC_Channel"=w132:i32, "Data.Config.Read message type"=w138:u16)
                    n71 = call "tsfifo_receive_flexray_msgs.vi"("Display message type"=w138, "AAPPChannel"=w132, "Path"=w131) -> ("error out"=w136:errorcluster, "return"=w139:i32, "FR_Buffer"=w133:T10[])  [unwired: 4 in, 1 out]
                    n72 = Equal To 0?(x=w139) -> (x = 0?=→"Receive Status":bool)
                    n73 = control-ref of="Receive_Data"() -> (w137:refnum<vi>)
                    n74 = call "FlexRay_FR_Tab.vi"("Fold Data"="Fold Data", "error in (no error)"=w136, "FR_Buffer"=w133, "FlexRay_Data IN"=w135, "MulticolumnListbox in"=w137) -> ("FlexRay_Data"=w134:T9)  [unwired: 6 in]
                  }
                  frame True {
                  }
                }
              }
            }
          }
          frame "DLL_PATH" {
            n75 = Variant To Data(type=path "" ("NewVal"), Variant=w146) -> (data=w143:path, error out=w142:errorcluster)  [unwired: 1 in]
            n76 = Bundle By Name(cluster=w147, "Data.Config.DLL_PATH"=w143, "error in"=w142) -> (w144:T9)
          }
          frame "Project_PATH" {
            n77 = Variant To Data(type=path "" ("NewVal"), Variant=w154) -> (data=w151:path, error out=w150:errorcluster)  [unwired: 1 in]
            n78 = Bundle By Name(cluster=w155, "Data.Config.Project_PATH"=w151, "error in"=w150) -> (w152:T9)
          }
          frame "BLF_Log_PATH" {
            n79 = Variant To Data(type=path "" ("NewVal"), Variant=w162) -> (data=w159:path, error out=w158:errorcluster)  [unwired: 1 in]
            n80 = Bundle By Name(cluster=w163, "Data.Config.BLF_Log_PATH"=w159, "error in"=w158) -> (w160:T9)
          }
          frame "XML Path" {
            n81 = Variant To Data(type=path "" ("NewVal"), Variant=w170) -> (data=w167:path, error out=w166:errorcluster)  [unwired: 1 in]
            n82 = Bundle By Name(cluster=w171, "Data.XML_Data.XML Path"=w167, "error in"=w166) -> (w168:T9)
          }
          frame "Read message type" {
            n83 = Variant To Data(type=u16 0, Variant=w178) -> (data=w176:u16, error out=w175:errorcluster)  [unwired: 1 in]
            n84 = Bundle By Name(cluster=w179, "Data.Config.Read message type"=w176, "error in"=w175) -> (w177:T9)
          }
          frame "Channel" {
            n85 = Variant To Data(type=0, Variant=w186) -> (data=w184:i32, error out=w183:errorcluster)  [unwired: 1 in]
            n86 = Bundle By Name(cluster=w187, "Data.Config.Channel"=w184, "error in"=w183) -> (w185:T9)
          }
          frame "XML loading channel" {
            n87 = Variant To Data(type=0, Variant=w194) -> (data=w192:i32, error out=w191:errorcluster)  [unwired: 1 in]
            n88 = Bundle By Name(cluster=w195, "Data.XML_Data.XML loading channel"=w192, "error in"=w191) -> (w193:T9)
          }
          frame "REC_Channel" {
            n89 = Variant To Data(type=0, Variant=w202) -> (data=w200:i32, error out=w199:errorcluster)  [unwired: 1 in]
            n90 = Bundle By Name(cluster=w203, "Data.Config.REC_Channel"=w200, "error in"=w199) -> (w201:T9)
          }
          frame "CycleNumber" {
            n91 = Variant To Data(type=u8 0, Variant=w210) -> (data=w208:u8, error out=w207:errorcluster)  [unwired: 1 in]
            n92 = Bundle By Name(cluster=w211, "Data.Config.CycleNumber"=w208, "error in"=w207) -> (w209:T9)
          }
          frame "ActualPayloadLength" {
            n93 = Variant To Data(type=u8 0, Variant=w218) -> (data=w216:u8, error out=w215:errorcluster)  [unwired: 1 in]
            n94 = Bundle By Name(cluster=w219, "Data.Config.ActualPayloadLength"=w216, "error in"=w215) -> (w217:T9)
          }
          frame "SlotId" {
            n95 = Variant To Data(type=u16 0, Variant=w226) -> (data=w224:u16, error out=w223:errorcluster)  [unwired: 1 in]
            n96 = Bundle By Name(cluster=w227, "Data.Config.SlotId"=w224, "error in"=w223) -> (w225:T9)
          }
          frame "ChannelMask" {
            n97 = Variant To Data(type=u16 0, Variant=w234) -> (data=w232:u16, error out=w231:errorcluster)  [unwired: 1 in]
            n98 = Bundle By Name(cluster=w235, "Data.Config.ChannelMask"=w232, "error in"=w231) -> (w233:T9)
          }
          frame "Send_Array" {
            n99 = Variant To Data(type=u8[] [] ("新值"), Variant=w242) -> (data=w240:u8[], error out=w239:errorcluster)  [unwired: 1 in]
            n100 = Bundle By Name(cluster=w243, "Data.Config.Send_Array"=w240, "error in"=w239) -> (w241:T9)
          }
          frame "Config update" {
            n101 = Variant To Data(type=w247, Variant=w248) -> (data=w249:T9, error out=w250:errorcluster)  [unwired: 1 in]
            n102 = Unbundle By Name(w249) -> ("Data"=w251:T18)
            n103 = Bundle By Name(cluster=w247, "Data"=w251, "error in"=w250) -> (w246:T9)
          }
          frame "Clear" {
            n104 = Bundle By Name(cluster=w257, "Data.FR_Frame_Buffer"=T10[] []) -> (w256:T9)
            n105 = property on="Receive_Data" class="MCListbox (严格)"("ItemNames"=string[][] [] ("项名")) -> ()  [unwired: 2 in, 2 out]
          }
          frame "Quit" {
          }
        }
        n106 = Unbundle By Name(w91) -> ("error in"=w90:errorcluster)
        n107 = Unbundle By Name(w94) -> ("message"=w93:string)
        n108 = call "error_collect.vi"("error in (no error)"=w90) -> ("error IO"=w88:errorcluster)  [unwired: 10 in]
        n109 = case shown="\"default\", 默认" w93 {
          tunnel: w100 -> [w111 w113]
          tunnel: w99 -> [w110 w112]
          tunnel: w94 -> [w109 _]
          tunnel: [w108 w113] -> w97
          tunnel: [w107 w112] -> w96
          frame "default", Default {
            n110 = Enqueue Element(queue=w111, element=w109, error in (no error)=w110) -> (queue out=w108:refnum<queue>, error out=w107:errorcluster)  [unwired: 1 in, 1 out]
          }
          frame "" {
          }
        }
        n111 = Bundle By Name(cluster=w91, "error in"=w88) -> (w89:T9)
      }
      n112 = while {
        tunnel: w86 -> [w285]
        tunnel: w82 -> [w284]
        tunnel: [w277] -> w85
        tunnel: [w276] -> w84
        shift-right: [w268] -> w76
        shift-left: w81 -> [w272]
        tunnel: w78 -> [w271]
        tunnel: w72 -> [w266]
        tunnel: w71 -> [w265]
        stop <- w275 stop-if-true
        # "Message Handling Loop"
        n113 = Dequeue Element(queue=w285, error in (no error)=w284) -> (queue out=w282:refnum<queue>, element=w283:T15, error out=w281:errorcluster)  [unwired: 1 in, 1 out]
        n114 = Unbundle By Name(w283) -> ("message"=w264:string, "data"=w278:variant)
        n115 = case shown="\"XML_Define\"" w264 {
          selector: w264 -> [_ _ w359 w380 w402 w424 w446 w468 w490 _ _ _ w863 w885 w907 w929 w951 w974 w996 w1012 w1034 _ w1098 _ w1137 _ _ _ _ _ _ _ _]
          tunnel: [w299 w330 w378 w400 w422 w444 w466 w488 w510 w547 w564 w857 w883 w905 w927 w949 w971 w993 w1007 w1023 w1051 w1062 w1107 w1129 w1145 w1156 w1180 w1193 w1204 w1216 w1243 w1260 w1284] -> w280
          tunnel: w282 -> [w299 w330 w378 w400 w422 w444 w466 w488 w510 w547 w564 w857 w883 w905 w927 w949 w971 w993 w1007 w1023 w1051 w1062 w1107 w1129 w1145 w1156 w1180 w1193 w1204 w1216 w1243 w1260 w1283]
          tunnel: w281 -> [w298 w329 w377 w399 w421 w443 w465 w487 w509 w546 w563 w856 w882 w904 w926 w948 w970 w992 w1006 w1022 w1050 w1061 w1106 w1128 w1144 w1155 w1179 w1192 w1203 w1215 w1242 w1259 w1281]
          tunnel: [w298 w329 w377 w399 w421 w443 w465 w487 w509 w546 w563 w856 w882 w904 w926 w948 w970 w992 w1006 w1022 w1050 w1061 w1106 w1128 w1144 w1155 w1179 w1192 w1203 w1215 w1242 w1259 w1282] -> w279
          tunnel: w278 -> [_ _ w376 w388 w410 w432 w455 w476 w498 _ w559 _ w871 w893 w915 w937 w959 w982 w1005 w1021 _ w1052 w1099 w1126 _ w1154 w1177 _ _ _ _ _ _]
          tunnel: [_ _ _ _ _ _ _ _ _ _ _ _ _ _ _ _ _ _ _ _ _ _ _ _ _ _ _ _ _ _ _ _ TRUE] -> w275
          tunnel: [w296 _ _ _ _ _ _ _ _ _ _ _ _ _ _ _ _ _ _ _ _ _ _ _ _ _ _ _ _ w1207 _ _ _] -> w274
          tunnel: [w293 w324 w365 w386 w408 w430 w453 w474 w496 w522 w551 w835 w869 w891 w913 w935 w957 w980 w995 w1009 w1039 w1057 w1102 w1124 w1136 w1151 w1175 w1181 w1194 w1205 w1238 w1258 w1274] -> w270
          tunnel: w272 -> [w293 w328 w368 w387 w409 w431 w454 w475 w497 w545 w551 w835 w870 w892 w914 w936 w958 w981 w995 w1009 w1049 w1060 w1105 w1127 w1143 w1150 w1178 w1182 w1195 w1209 w1238 w1258 w1261]
          tunnel: w271 -> [_ _ _ _ _ _ _ _ _ _ _ _ _ _ _ _ _ _ w999 w1013 _ _ _ _ _ _ _ _ _ _ _ _ w1280]
          tunnel: w266 -> [_ _ w363 w382 w404 w426 w448 w470 w492 w534 _ w844 w865 w887 w909 w931 w953 w976 _ _ _ _ _ _ w1131 _ _ _ _ _ _ _ w1279]
          tunnel: w265 -> [_ _ w362 w381 w403 w425 w447 w469 w491 w532 _ w843 w864 w886 w908 w930 w952 w975 _ _ _ _ _ _ w1130 _ _ _ _ _ _ _ w1278]
          frame "eee", Default {
            w294 = ""
            n116 = Bundle By Name(cluster=T15 {"Sender"="", "receiver"="", "message"="", "data"=variant} ("Communication message"), "Sender"=w294, "receiver"=w294, "message"=w294, "data"=variant) -> (w296:T15)
          }
          frame "Init" {
            n117 = Unbundle By Name(w328) -> ("Data.Config.DLL_PATH"=w327:path, "Communication message.Sender"=w326:string, "Data.Config.Project_PATH"=w325:path)
            n118 = call "initialize_lib_tsmaster_with_project.vi"("projectfile"=w325, "AppName"=w326, "Path input"=w327) -> ("error output"=w307:errorcluster, "Path output"=w317:path)  [unwired: 7 in]
            n119 = call "tsapp_disconnect.vi"("error in (no error)"=w307, "Path"=w317) -> ("error output"=w318:errorcluster, "retuen"=w315:i32, "Path output"=w316:path)  [unwired: 7 in]
            n120 = call "Device_Detection.vi"("error in (no error)"=w318, "Path"=w316) -> ("error out"=w309:errorcluster, "retuen"=w314:i32, "Path output"=w310:path)  [unwired: 7 in]
            n121 = flat-sequence {
              tunnel: w310 -> [w351]
              tunnel: w309 -> [w350]
              tunnel: [w351] -> w322
              tunnel: [w350] -> w321
              tunnel: [w354] -> w319
              tunnel: [w356] -> w320
              tunnel: w322 -> [w356]
              tunnel: w321 -> [w355]
              frame #0 {
                n122 = Wait (ms)(milliseconds to wait=u32 500) -> ()  [unwired: 1 out]
              }
              frame #1 {
                n123 = call <vilib>:"Set Busy.vi"("error in (no error)"=w355, "disable click? (T)"=TRUE) -> ("error out"=w354:errorcluster)  [unwired: 8 in, 1 out]
              }
            }
            n124 = case shown="真" "TS_Mapping" {
              tunnel: w320 -> [w339 w344]
              tunnel: w319 -> [w338 w343]
              tunnel: [w339 w342] -> w305
              tunnel: [_ w341] -> w312
              tunnel: [w338 w340] -> w303
              frame False {
              }
              frame True {
                n125 = call "tsapp_show_hardware_configuration_window.vi"("error in (no error)"=w343, "路径输入"=w344) -> ("error out"=w340:errorcluster, "function return"=w341:i32, "路径输出"=w342:path)  [unwired: 7 in]
              }
            }
            n126 = case shown="真" "CH_Mapping" {
              tunnel: w305 -> [w332 w337]
              tunnel: w303 -> [w331 w335]
              tunnel: [w332 w336] -> w304
              tunnel: [_ w333] -> w301
              tunnel: [w331 w334] -> w302
              frame False {
              }
              frame True {
                n127 = call "tsapp_show_channel_mapping_window.vi"("error in (no error)"=w335, "路径输入"=w337) -> ("error out"=w334:errorcluster, "function return"=w333:i32, "路径输出"=w336:path)  [unwired: 7 in]
              }
            }
            n128 = Build Array(w315, w314, w312, w301) -> (w313:i32[])
            n129 = call <vilib>:"Unset Busy.vi"("error in (no error)"=w302) -> ("error out"=w308:errorcluster)  [unwired: 10 in]
            n130 = for {
              tunnel: w304 -> [w347]
              shift-right: [w348] -> w323
              shift-left: w308 -> [w349]
              tunnel: w313 -> [w346] mode=indexing
              tunnel: string[] ["DisConnect", "Dete", "Show Config", "Show Mapping"] -> [w345] mode=indexing
              n131 = call "error_display.vi"("error in"=w349, "Action name"=w345, "return"=w346, "DLL path"=w347) -> ("error out"=w348:errorcluster)  [unwired: 6 in, 1 out]
            }
            n132 = Bundle By Name(cluster=w328, "error in"=w323) -> (w324:T9)
          }
          frame "DLL_PATH" {
            n133 = Variant To Data(type=path "" ("NewVal"), Variant=w376) -> (data=w357:path, error out=w369:errorcluster)  [unwired: 1 in]
            n134 = Unbundle By Name(w368) -> ("Communication message.Sender"=w367:string)
            n135 = Current VI's Path() -> (path=w374:path)
            n136 = Strip Path(path=w374) -> (stripped path=w370:path)  [unwired: 1 out]
            n137 = Bundle By Name(cluster=w368, "Data.Config.DLL_PATH"=w357) -> (w366:T9)
            n138 = Build Path(base path=w370, name or relative path="data") -> (appended path=w373:path)
            n139 = call "FlexRay_Configuration_Save.vi"("path"=w373, "error in (no error)"=w369, "Config Name"=w367, "Read/Write"=enum16{"Read", "Write"}."Write", "FlexRay_Data"=w366) -> ("error in (no error)"=w364:errorcluster)  [unwired: 4 in, 2 out]
            n140 = Bundle By Name(cluster=w366, "error in"=w364) -> (w365:T9)
            n141 = To Variant(anything=w357) -> (Variant=w358:variant)
            n142 = Bundle By Name(cluster=T15 {"Sender"="", "receiver"="", "message"="", "data"=variant} ("元素"), "message"=w359, "data"=w358) -> (w360:T15)
            n143 = Enqueue Element(queue=w363, element=w360, error in (no error)=w362) -> ()  [unwired: 1 in, 3 out]
          }
          frame "Project_PATH" {
            n144 = Variant To Data(type=path "" ("NewVal"), Variant=w388) -> (data=w379:path, error out=w392:errorcluster)  [unwired: 1 in]
            n145 = Unbundle By Name(w387) -> ("Communication message.Sender"=w391:string)
            n146 = Current VI's Path() -> (path=w397:path)
            n147 = Strip Path(path=w397) -> (stripped path=w393:path)  [unwired: 1 out]
            n148 = Bundle By Name(cluster=w387, "Data.Config.Project_PATH"=w379) -> (w390:T9)
            n149 = Build Path(base path=w393, name or relative path="data") -> (appended path=w396:path)
            n150 = call "FlexRay_Configuration_Save.vi"("path"=w396, "error in (no error)"=w392, "Config Name"=w391, "Read/Write"=enum16{"Read", "Write"}."Write", "FlexRay_Data"=w390) -> ("error in (no error)"=w389:errorcluster)  [unwired: 4 in, 2 out]
            n151 = Bundle By Name(cluster=w390, "error in"=w389) -> (w386:T9)
            n152 = To Variant(anything=w379) -> (Variant=w383:variant)
            n153 = Bundle By Name(cluster=T15 {"Sender"="", "receiver"="", "message"="", "data"=variant} ("元素"), "message"=w380, "data"=w383) -> (w384:T15)
            n154 = Enqueue Element(queue=w382, element=w384, error in (no error)=w381) -> ()  [unwired: 1 in, 3 out]
          }
          frame "BLF_Log_PATH" {
            n155 = Variant To Data(type=path "" ("NewVal"), Variant=w410) -> (data=w401:path, error out=w414:errorcluster)  [unwired: 1 in]
            n156 = Unbundle By Name(w409) -> ("Communication message.Sender"=w413:string)
            n157 = Current VI's Path() -> (path=w419:path)
            n158 = Strip Path(path=w419) -> (stripped path=w415:path)  [unwired: 1 out]
            n159 = Bundle By Name(cluster=w409, "Data.Config.BLF_Log_PATH"=w401) -> (w412:T9)
            n160 = Build Path(base path=w415, name or relative path="data") -> (appended path=w418:path)
            n161 = call "FlexRay_Configuration_Save.vi"("path"=w418, "error in (no error)"=w414, "Config Name"=w413, "Read/Write"=enum16{"Read", "Write"}."Write", "FlexRay_Data"=w412) -> ("error in (no error)"=w411:errorcluster)  [unwired: 4 in, 2 out]
            n162 = Bundle By Name(cluster=w412, "error in"=w411) -> (w408:T9)
            n163 = To Variant(anything=w401) -> (Variant=w405:variant)
            n164 = Bundle By Name(cluster=T15 {"Sender"="", "receiver"="", "message"="", "data"=variant} ("元素"), "message"=w402, "data"=w405) -> (w406:T15)
            n165 = Enqueue Element(queue=w404, element=w406, error in (no error)=w403) -> ()  [unwired: 1 in, 3 out]
          }
          frame "XML Path" {
            n166 = Variant To Data(type=path "" ("NewVal"), Variant=w432) -> (data=w423:path, error out=w436:errorcluster)  [unwired: 1 in]
            n167 = Unbundle By Name(w431) -> ("Communication message.Sender"=w435:string)
            n168 = Current VI's Path() -> (path=w441:path)
            n169 = Strip Path(path=w441) -> (stripped path=w437:path)  [unwired: 1 out]
            n170 = Bundle By Name(cluster=w431, "Data.XML_Data.XML Path"=w423) -> (w434:T9)
            n171 = Build Path(base path=w437, name or relative path="data") -> (appended path=w440:path)
            n172 = call "FlexRay_Configuration_Save.vi"("path"=w440, "error in (no error)"=w436, "Config Name"=w435, "Read/Write"=enum16{"Read", "Write"}."Write", "FlexRay_Data"=w434) -> ("error in (no error)"=w433:errorcluster)  [unwired: 4 in, 2 out]
            n173 = Bundle By Name(cluster=w434, "error in"=w433) -> (w430:T9)
            n174 = To Variant(anything=w423) -> (Variant=w427:variant)
            n175 = Bundle By Name(cluster=T15 {"Sender"="", "receiver"="", "message"="", "data"=variant} ("元素"), "message"=w424, "data"=w427) -> (w428:T15)
            n176 = Enqueue Element(queue=w426, element=w428, error in (no error)=w425) -> ()  [unwired: 1 in, 3 out]
          }
          frame "Read message type" {
            n177 = Variant To Data(type=u16 0, Variant=w455) -> (data=w445:u16, error out=w459:errorcluster)  [unwired: 1 in]
            n178 = Unbundle By Name(w454) -> ("Communication message.Sender"=w458:string)
            n179 = Current VI's Path() -> (path=w464:path)
            n180 = Strip Path(path=w464) -> (stripped path=w460:path)  [unwired: 1 out]
            n181 = Bundle By Name(cluster=w454, "Data.Config.Read message type"=w445) -> (w457:T9)
            n182 = Build Path(base path=w460, name or relative path="data") -> (appended path=w463:path)
            n183 = call "FlexRay_Configuration_Save.vi"("path"=w463, "error in (no error)"=w459, "Config Name"=w458, "Read/Write"=enum16{"Read", "Write"}."Write", "FlexRay_Data"=w457) -> ("error in (no error)"=w456:errorcluster)  [unwired: 4 in, 2 out]
            n184 = Bundle By Name(cluster=w457, "error in"=w456) -> (w453:T9)
            n185 = To Variant(anything=w445) -> (Variant=w449:variant)
            n186 = Bundle By Name(cluster=T15 {"Sender"="", "receiver"="", "message"="", "data"=variant} ("元素"), "message"=w446, "data"=w449) -> (w450:T15)
            n187 = Enqueue Element(queue=w448, element=w450, error in (no error)=w447) -> ()  [unwired: 1 in, 3 out]
          }
          frame "Channel" {
            n188 = Variant To Data(type=0, Variant=w476) -> (data=w467:i32, error out=w481:errorcluster)  [unwired: 1 in]
            n189 = Unbundle By Name(w475) -> ("Communication message.Sender"=w480:string)
            n190 = Current VI's Path() -> (path=w486:path)
            n191 = Strip Path(path=w486) -> (stripped path=w482:path)  [unwired: 1 out]
            n192 = Bundle By Name(cluster=w475, "Data.Config.Channel"=w467) -> (w479:T9)
            n193 = Build Path(base path=w482, name or relative path="data") -> (appended path=w485:path)
            n194 = call "FlexRay_Configuration_Save.vi"("path"=w485, "error in (no error)"=w481, "Config Name"=w480, "Read/Write"=enum16{"Read", "Write"}."Write", "FlexRay_Data"=w479) -> ("error in (no error)"=w478:errorcluster)  [unwired: 4 in, 2 out]
            n195 = Bundle By Name(cluster=w479, "error in"=w478) -> (w474:T9)
            n196 = To Variant(anything=w467) -> (Variant=w471:variant)
            n197 = Bundle By Name(cluster=T15 {"Sender"="", "receiver"="", "message"="", "data"=variant} ("元素"), "message"=w468, "data"=w471) -> (w472:T15)
            n198 = Enqueue Element(queue=w470, element=w472, error in (no error)=w469) -> ()  [unwired: 1 in, 3 out]
          }
          frame "XML loading channel" {
            n199 = Variant To Data(type=0, Variant=w498) -> (data=w489:i32, error out=w503:errorcluster)  [unwired: 1 in]
            n200 = Unbundle By Name(w497) -> ("Communication message.Sender"=w502:string)
            n201 = Current VI's Path() -> (path=w508:path)
            n202 = Strip Path(path=w508) -> (stripped path=w504:path)  [unwired: 1 out]
            n203 = Bundle By Name(cluster=w497, "Data.XML_Data.XML loading channel"=w489) -> (w501:T9)
            n204 = Build Path(base path=w504, name or relative path="data") -> (appended path=w507:path)
            n205 = call "FlexRay_Configuration_Save.vi"("path"=w507, "error in (no error)"=w503, "Config Name"=w502, "Read/Write"=enum16{"Read", "Write"}."Write", "FlexRay_Data"=w501) -> ("error in (no error)"=w500:errorcluster)  [unwired: 4 in, 2 out]
            n206 = Bundle By Name(cluster=w501, "error in"=w500) -> (w496:T9)
            n207 = To Variant(anything=w489) -> (Variant=w493:variant)
            n208 = Bundle By Name(cluster=T15 {"Sender"="", "receiver"="", "message"="", "data"=variant} ("元素"), "message"=w490, "data"=w493) -> (w494:T15)
            n209 = Enqueue Element(queue=w492, element=w494, error in (no error)=w491) -> ()  [unwired: 1 in, 3 out]
          }
          frame "Load_XML" {
            n210 = Unbundle By Name(w545) -> ("Data.DataBase_array"=w511:T12, "Data.Config.DLL_PATH"=w544:path, "Data.XML_Data.XML Path"=w543:path, "Data.XML_Data.XML loading channel"=w542:i32)
            n211 = Build Array(w542) -> (w541:i32[])
            n212 = control-ref of="Tree control"() -> (w539:refnum<vi>)
            n213 = call "FlexRay_XML_Load.vi"("DataBase_array"=w511, "Channels"=w541, "XML Path"=w543, "DLL_PATH"=w544) -> ("error out"=w540:errorcluster, "result"=w537:bool)  [unwired: 6 in]
            "Laod XML Successful?" <- w537
            n214 = call "FlexRay_DBTableToTree.vi"("error in (no error)"=w540, "DataBase_array"=w511, "reference"=w539) -> ("error out"=w513:errorcluster)  [unwired: 8 in]
            n215 = call "Message signal name resolution.vi"("error in (no error)"=w513, "BusType"=enum16{"LIN", "FlexRay"}."FlexRay", "DataBase_array"=w511) -> ("error out"=w512:errorcluster, "Signals Name array"=w527:string[][], "Frame Name array"=w525:string[])  [unwired: 6 in]
            n216 = Bundle By Name(cluster=w545, "error in"=w512) -> (w522:T9)
            n217 = case shown="假" w537 {
              tunnel: ["Load_XML fail " ("消息") "Load_XML successful " ("消息")] -> w538
              frame False {
              }
              frame True {
              }
            }
            n218 = Index Array(array=w527) -> (element=w529:string[])  [unwired: 2 in]
            n219 = property on="Messages" class="CmbBox"("Strings[]"=w525) -> ()  [unwired: 2 in, 2 out]
            n220 = Build Array(w529, string[] [] ("元素")) -> (w526:string[][])
            n221 = Index Array(array=w525) -> (element=w523:string)  [unwired: 1 in]
            n222 = call "FlexRay_Match_Message.vi"("DataBase_array"=w511, "Message"=w523) -> ("Frame"=w524:T17)  [unwired: 9 in]
            n223 = Unbundle By Name(w524) -> ("Frame_Properties.FFRSlotId"=w519:u16, "Frame_Properties.FFRDLC"=w518:u16, "Frame_Properties.FFRChannelMask"=w517:u8, "Frame_Properties.FFRBaseCycle"=w516:u8, "Frame_Properties.FFRCycleRepetition"=w515:u8, "signal_array"=w521:T5[])
            n224 = Add(x=w516, y=w515) -> (x+y=w514:u8)
            n225 = local write "SlotId"(w519) -> ()
            n226 = local write "ActualPayloadLength"(w518) -> ()
            n227 = local write "ChannelMask"(w517) -> ()
            n228 = call "Signal_Name_Conver.vi"("signal_array"=w521) -> ("Signals"=w520:string[][])  [unwired: 10 in]
            n229 = local write "Signals"(w520) -> ()
            n230 = local write "CycleNumber"(w514) -> ()
            n231 = local write "Signals"(w526) -> ()
            n232 = To Variant(anything=w522) -> (Variant=w535:variant)
            n233 = property on="Messages" class="CmbBox"("Value"=w523) -> ()  [unwired: 2 in, 2 out]
            n234 = Bundle By Name(cluster=T15 {"Sender"="", "receiver"="", "message"="", "data"=variant} ("Communication message"), "message"="Config update" ("Communication message.message"), "data"=w535) -> (w531:T15)
            n235 = call "Log.vi"("Data"=w538) -> ()  [unwired: 3 in]
            n236 = One Button Dialog(message=w538) -> ()  [unwired: 1 in, 1 out]
            n237 = Enqueue Element(queue=w534, element=w531, error in (no error)=w532) -> ()  [unwired: 1 in, 3 out]
          }
          frame "XML_Define" {
            n238 = Variant To Data(type=refnum<vi> refnum ("CtlRef"), Variant=w559) -> (data=w558:refnum<vi>)  [unwired: 1 in, 1 out]
            n239 = property class="Tree (严格)"(reference=w558) -> (reference out=w561:refnum<vi>, error out=w560:errorcluster, "Value"=w552:string)  [unwired: 1 in]
            n240 = Unbundle By Name(w551) -> ("Data.DataBase_array"=w550:T12)
            n241 = invoke class="Tree (严格)" method="Navigate Tree.Get Parent"(reference=w561, error in=w560, "tag"=w552) -> (reference out=w555:refnum<vi>, error out=w554:errorcluster, "Navigate Tree:Get Parent"=w553:string)  [unwired: 1 in, 1 out]
            n242 = xnode "匹配正则表达式"("输入字符串"=w553, "正则表达式"="_[0-9]+$" ("regular expression")) -> ("匹配之前"=w556:string)  [unwired: 4 in, 4 out]
            n243 = case shown="\"Messages\", \"RX Message\", \"TX Message\"" w556 {
              tunnel: w555 -> [w571 _]
              tunnel: w554 -> [w570 w589]
              tunnel: w553 -> [w569 _]
              tunnel: w552 -> [w567 w599]
              tunnel: w550 -> [w565 w587]
              frame Default {
                n244 = invoke class="Tree (严格)" method="Navigate Tree.Get Parent"(reference=w571, error in=w570, "tag"=w569) -> (error out=w572:errorcluster, "Navigate Tree:Get Parent"=w573:string)  [unwired: 1 in, 2 out]
                n245 = call <vilib>:"Clear Errors.vi"("error in (no error)"=w572) -> ("error out"=w566:errorcluster)  [unwired: 5 in, 1 out]
                n246 = Equal?(x=w573, y="Messages") -> (x = y?=w568:bool)
                n247 = case shown="真" w568 {
                  tunnel: w567 -> [_ w582]
                  tunnel: w566 -> [_ w578]
                  tunnel: w565 -> [_ w575]
                  frame False {
                  }
                  frame True {
                    n248 = control-ref of="Signal Table"() -> (w586:refnum<vi>)
                    n249 = call "FlexRay_Match_Signal.vi"("DataBase_array"=w575, "Signal"=w582) -> ("TDBSignalProperties"=w581:T5)  [unwired: 9 in]
                    n250 = control-ref of="XML Tab"() -> (w584:refnum<vi>)
                    n251 = property on="Property Node" class="TabCtl (严格)"(reference=w584, error in=w578, "Value"=enum32{"Message", "Signal"}."Signal" ("值")) -> (error out=w577:errorcluster)  [unwired: 1 out]
                    n252 = property on="Property Node" class="Tbl (严格)"(reference=w586, error in=w577) -> (reference out=w585:refnum<vi>, error out=w576:errorcluster, "Value"=w580:string[][])
                    n253 = call "FlexRay_Signal analysis.vi"("TDBSignalProperties"=w581, "Value in"=w580) -> ("Value out"=w579:string[][])  [unwired: 9 in]
                    n254 = property on="Property Node" class="Tbl (严格)"(reference=w585, error in=w576, "Value"=w579) -> ()  [unwired: 2 out]
                  }
                }
              }
              frame "Messages", "RX Message", "TX Message" {
                n255 = control-ref of="Message Table"() -> (w597:refnum<vi>)
                n256 = control-ref of="XML Tab"() -> (w591:refnum<vi>)
                n257 = xnode "匹配正则表达式"("输入字符串"=w599, "正则表达式"="_[0-9]+$" ("regular expression")) -> ("匹配之前"=w598:string)  [unwired: 4 in, 4 out]
                n258 = call "FlexRay_Match_Message.vi"("DataBase_array"=w587, "Message"=w598) -> ("Frame"=w593:T17)  [unwired: 9 in]
                n259 = property on="Property Node" class="TabCtl (严格)"(reference=w591, error in=w589, "Value"=enum32{"Message", "Signal"}."Message" ("值")) -> (error out=w588:errorcluster)  [unwired: 1 out]
                n260 = property on="Property Node" class="Tbl (严格)"(reference=w597, error in=w588) -> (reference out=w596:refnum<vi>, error out=w595:errorcluster, "Value"=w594:string[][])
                n261 = call "FlexRay_Message analysis.vi"("Frame"=w593, "Value in"=w594) -> ("Value out"=w592:string[][])  [unwired: 9 in]
                n262 = property on="Property Node" class="Tbl (严格)"(reference=w596, error in=w595, "Value"=w592) -> ()  [unwired: 2 out]
              }
            }
          }
          frame "Unload" {
            n263 = Unbundle By Name(w835) -> ("Data.Config.DLL_PATH"=w855:path)
            n264 = Unbundle By Name(w835) -> ("Data.DataBase_array"=w837:T12)
            n265 = property on="Messages" class="CmbBox"("Strings[]"=string[] [] ("字符串[]")) -> (error out=w841:errorcluster)  [unwired: 2 in, 1 out]
            n266 = local write "Signals"(string[][] [] ("Signals")) -> ()
            n267 = call "tsdb_unload_flexray_dbs.vi"("路径输入"=w855) -> ("error out"=w851:errorcluster, "function return"=w850:i32)  [unwired: 8 in, 1 out]
            n268 = Unbundle By Name(w851) -> ("status"=w854:bool)
            n269 = Equal To 0?(x=w850) -> (x = 0?=w853:bool)
            n270 = property on="Messages" class="CmbBox"(error in=w841, "Value"="" ("Messages")) -> ()  [unwired: 1 in, 2 out]
            n271 = Not(x=w854) -> (.not. x?=w852:bool)
            n272 = property class="Arr (严格)"(reference=w837, "Value"=T1 [] ("值")) -> ()  [unwired: 1 in, 2 out]
            n273 = Compound Arithmetic op=AND(w853, w852) -> (w849:bool)
            n274 = case shown="真" w849 {
              tunnel: ["Unload_XML fail " ("消息") "Unload_XML successful " ("消息")] -> w848
              frame False {
              }
              frame True {
                n275 = control-ref of="Tree control"() -> (w861:refnum<vi>)
                n276 = invoke class="Tree (严格)" method="Edit Tree Items.Delete"(reference=w861) -> ()  [unwired: 4 in, 5 out]
                n277 = local write "Laod XML Successful?"(FALSE ("Laod XML Successful?")) -> ()
              }
            }
            n278 = To Variant(anything=w835) -> (Variant=w846:variant)
            n279 = Bundle By Name(cluster=T15 {"Sender"="", "receiver"="", "message"="", "data"=variant} ("Communication message"), "message"="Config update" ("Communication message.message"), "data"=w846) -> (w845:T15)
            n280 = One Button Dialog(message=w848) -> ()  [unwired: 1 in, 1 out]
            n281 = call "Log.vi"("Data"=w848) -> ()  [unwired: 3 in]
            n282 = Enqueue Element(queue=w844, element=w845, error in (no error)=w843) -> ()  [unwired: 1 in, 3 out]
          }
          frame "REC_Channel" {
            n283 = Variant To Data(type=0, Variant=w871) -> (data=w862:i32, error out=w876:errorcluster)  [unwired: 1 in]
            n284 = Unbundle By Name(w870) -> ("Communication message.Sender"=w875:string)
            n285 = Current VI's Path() -> (path=w881:path)
            n286 = Strip Path(path=w881) -> (stripped path=w877:path)  [unwired: 1 out]
            n287 = Bundle By Name(cluster=w870, "Data.Config.REC_Channel"=w862) -> (w874:T9)
            n288 = Build Path(base path=w877, name or relative path="data") -> (appended path=w880:path)
            n289 = call "FlexRay_Configuration_Save.vi"("path"=w880, "error in (no error)"=w876, "Config Name"=w875, "Read/Write"=enum16{"Read", "Write"}."Write", "FlexRay_Data"=w874) -> ("error in (no error)"=w873:errorcluster)  [unwired: 4 in, 2 out]
            n290 = Bundle By Name(cluster=w874, "error in"=w873) -> (w869:T9)
            n291 = To Variant(anything=w862) -> (Variant=w866:variant)
            n292 = Bundle By Name(cluster=T15 {"Sender"="", "receiver"="", "message"="", "data"=variant} ("元素"), "message"=w863, "data"=w866) -> (w867:T15)
            n293 = Enqueue Element(queue=w865, element=w867, error in (no error)=w864) -> ()  [unwired: 1 in, 3 out]
          }
          frame "CycleNumber" {
            n294 = Variant To Data(type=u8 0, Variant=w893) -> (data=w884:u8, error out=w898:errorcluster)  [unwired: 1 in]
            n295 = Unbundle By Name(w892) -> ("Communication message.Sender"=w897:string)
            n296 = Current VI's Path() -> (path=w903:path)
            n297 = Strip Path(path=w903) -> (stripped path=w899:path)  [unwired: 1 out]
            n298 = Bundle By Name(cluster=w892, "Data.Config.CycleNumber"=w884) -> (w896:T9)
            n299 = Build Path(base path=w899, name or relative path="data") -> (appended path=w902:path)
            n300 = call "FlexRay_Configuration_Save.vi"("path"=w902, "error in (no error)"=w898, "Config Name"=w897, "Read/Write"=enum16{"Read", "Write"}."Write", "FlexRay_Data"=w896) -> ("error in (no error)"=w895:errorcluster)  [unwired: 4 in, 2 out]
            n301 = Bundle By Name(cluster=w896, "error in"=w895) -> (w891:T9)
            n302 = To Variant(anything=w884) -> (Variant=w888:variant)
            n303 = Bundle By Name(cluster=T15 {"Sender"="", "receiver"="", "message"="", "data"=variant} ("元素"), "message"=w885, "data"=w888) -> (w889:T15)
            n304 = Enqueue Element(queue=w887, element=w889, error in (no error)=w886) -> ()  [unwired: 1 in, 3 out]
          }
          frame "ActualPayloadLength" {
            n305 = Variant To Data(type=u8 0, Variant=w915) -> (data=w906:u8, error out=w920:errorcluster)  [unwired: 1 in]
            n306 = Unbundle By Name(w914) -> ("Communication message.Sender"=w919:string)
            n307 = Current VI's Path() -> (path=w925:path)
            n308 = Strip Path(path=w925) -> (stripped path=w921:path)  [unwired: 1 out]
            n309 = Bundle By Name(cluster=w914, "Data.Config.ActualPayloadLength"=w906) -> (w918:T9)
            n310 = Build Path(base path=w921, name or relative path="data") -> (appended path=w924:path)
            n311 = call "FlexRay_Configuration_Save.vi"("path"=w924, "error in (no error)"=w920, "Config Name"=w919, "Read/Write"=enum16{"Read", "Write"}."Write", "FlexRay_Data"=w918) -> ("error in (no error)"=w917:errorcluster)  [unwired: 4 in, 2 out]
            n312 = Bundle By Name(cluster=w918, "error in"=w917) -> (w913:T9)
            n313 = To Variant(anything=w906) -> (Variant=w910:variant)
            n314 = Bundle By Name(cluster=T15 {"Sender"="", "receiver"="", "message"="", "data"=variant} ("元素"), "message"=w907, "data"=w910) -> (w911:T15)
            n315 = Enqueue Element(queue=w909, element=w911, error in (no error)=w908) -> ()  [unwired: 1 in, 3 out]
          }
          frame "SlotId" {
            n316 = Variant To Data(type=u16 0, Variant=w937) -> (data=w928:u16, error out=w942:errorcluster)  [unwired: 1 in]
            n317 = Unbundle By Name(w936) -> ("Communication message.Sender"=w941:string)
            n318 = Current VI's Path() -> (path=w947:path)
            n319 = Strip Path(path=w947) -> (stripped path=w943:path)  [unwired: 1 out]
            n320 = Bundle By Name(cluster=w936, "Data.Config.SlotId"=w928) -> (w940:T9)
            n321 = Build Path(base path=w943, name or relative path="data") -> (appended path=w946:path)
            n322 = call "FlexRay_Configuration_Save.vi"("path"=w946, "error in (no error)"=w942, "Config Name"=w941, "Read/Write"=enum16{"Read", "Write"}."Write", "FlexRay_Data"=w940) -> ("error in (no error)"=w939:errorcluster)  [unwired: 4 in, 2 out]
            n323 = Bundle By Name(cluster=w940, "error in"=w939) -> (w935:T9)
            n324 = To Variant(anything=w928) -> (Variant=w932:variant)
            n325 = Bundle By Name(cluster=T15 {"Sender"="", "receiver"="", "message"="", "data"=variant} ("元素"), "message"=w929, "data"=w932) -> (w933:T15)
            n326 = Enqueue Element(queue=w931, element=w933, error in (no error)=w930) -> ()  [unwired: 1 in, 3 out]
          }
          frame "ChannelMask" {
            n327 = Variant To Data(type=u16 0, Variant=w959) -> (data=w950:u16, error out=w964:errorcluster)  [unwired: 1 in]
            n328 = Unbundle By Name(w958) -> ("Communication message.Sender"=w963:string)
            n329 = Current VI's Path() -> (path=w969:path)
            n330 = Strip Path(path=w969) -> (stripped path=w965:path)  [unwired: 1 out]
            n331 = Bundle By Name(cluster=w958, "Data.Config.ChannelMask"=w950) -> (w962:T9)
            n332 = Build Path(base path=w965, name or relative path="data") -> (appended path=w968:path)
            n333 = call "FlexRay_Configuration_Save.vi"("path"=w968, "error in (no error)"=w964, "Config Name"=w963, "Read/Write"=enum16{"Read", "Write"}."Write", "FlexRay_Data"=w962) -> ("error in (no error)"=w961:errorcluster)  [unwired: 4 in, 2 out]
            n334 = Bundle By Name(cluster=w962, "error in"=w961) -> (w957:T9)
            n335 = To Variant(anything=w950) -> (Variant=w954:variant)
            n336 = Bundle By Name(cluster=T15 {"Sender"="", "receiver"="", "message"="", "data"=variant} ("元素"), "message"=w951, "data"=w954) -> (w955:T15)
            n337 = Enqueue Element(queue=w953, element=w955, error in (no error)=w952) -> ()  [unwired: 1 in, 3 out]
          }
          frame "Send_Array" {
            n338 = Variant To Data(type=u8[] [] ("新值"), Variant=w982) -> (data=w973:u8[], error out=w986:errorcluster)  [unwired: 1 in]
            n339 = Unbundle By Name(w981) -> ("Communication message.Sender"=w985:string)
            n340 = Current VI's Path() -> (path=w991:path)
            n341 = Strip Path(path=w991) -> (stripped path=w987:path)  [unwired: 1 out]
            n342 = Bundle By Name(cluster=w981, "Data.Config.Send_Array"=w973) -> (w984:T9)
            n343 = Build Path(base path=w987, name or relative path="data") -> (appended path=w990:path)
            n344 = call "FlexRay_Configuration_Save.vi"("path"=w990, "error in (no error)"=w986, "Config Name"=w985, "Read/Write"=enum16{"Read", "Write"}."Write", "FlexRay_Data"=w984) -> ("error in (no error)"=w983:errorcluster)  [unwired: 4 in, 2 out]
            n345 = Bundle By Name(cluster=w984, "error in"=w983) -> (w980:T9)
            n346 = To Variant(anything=w973) -> (Variant=w977:variant)
            n347 = Bundle By Name(cluster=T15 {"Sender"="", "receiver"="", "message"="", "data"=variant} ("元素"), "message"=w974, "data"=w977) -> (w978:T15)
            n348 = Enqueue Element(queue=w976, element=w978, error in (no error)=w975) -> ()  [unwired: 1 in, 3 out]
          }
          frame "Messages" {
            w1001 = T15 {"Sender"="", "receiver"="", "message"="", "data"=variant}  # Message
            n349 = Unbundle By Name(w995) -> ("Data.DataBase_array"=w994:T12)
            n350 = Variant To Data(type=w996, Variant=w1005) -> (data=w1002:string)  [unwired: 1 in, 1 out]
            n351 = call "FlexRay_Match_Message.vi"("DataBase_array"=w994, "Message"=w1002) -> ("Frame"=w998:T17)  [unwired: 9 in]
            n352 = Unbundle By Name(w998) -> ("signal_array"=w1004:T5[])
            n353 = call "Signal_Name_Conver.vi"("signal_array"=w1004) -> ("Signals"=w1003:string[][])  [unwired: 10 in]
            n354 = local write "Signals"(w1003) -> ()
            n355 = To Variant(anything=w998) -> (Variant=w997:variant)
            n356 = Bundle By Name(cluster=w1001, "message"=w996, "data"=w997) -> (w1000:T15)
            n357 = Generate User Event(user event=w999, event data cluster=w1000) -> ()  [unwired: 2 in, 2 out]
          }
          frame "Signals" {
            w1015 = T15 {"Sender"="", "receiver"="", "message"="", "data"=variant}  # Message
            n358 = local read "ActualPayloadLength"() -> (w1018:u8)
            n359 = Variant To Data(type=string[][] [] ("新值"), Variant=w1021) -> (data=w1019:string[][])  [unwired: 1 in, 1 out]
            n360 = Transpose 2D Array(2D array=w1019) -> (transposed array=w1017:string[][])
            n361 = Unbundle By Name(w1009) -> ("Data.DataBase_array"=w1008:T12)
            n362 = for {
              N: w1018 -> [_]
              tunnel: [u8 0] -> w1016 mode=indexing
            }
            n363 = for {
              tunnel: w1017 -> [w1032] mode=indexing
              shift-right: [w1026] -> w1010
              shift-left: w1016 -> [w1025]
              tunnel: w1008 -> [w1024]
              n364 = Index Array(array=w1032) -> (element #1=w1030:string, element #2=w1031:string)  [unwired: 2 in]
              n365 = Fract/Exp String To Number(string=w1031) -> (number=w1027:dbl)  [unwired: 3 in, 1 out]
              n366 = call "FlexRay_Match_Signal.vi"("DataBase_array"=w1024, "Signal"=w1030) -> ("TDBSignalProperties"=w1029:T5)  [unwired: 9 in]
              n367 = Unbundle By Name(w1029) -> ("TFlexRaySignal"=w1028:T8)
              n368 = call "FlexRay_SignalValue_Conver_Raw.vi"("Signal_Value"=w1027, "TFlexRaySignal"=w1028, "data in"=w1025) -> ("data"=w1026:u8[])  [unwired: 8 in]
            }
            n369 = To Variant(anything=w1010) -> (Variant=w1011:variant)
            n370 = Bundle By Name(cluster=w1015, "message"=w1012, "data"=w1011) -> (w1014:T15)
            n371 = Generate User Event(user event=w1013, event data cluster=w1014) -> ()  [unwired: 2 in, 2 out]
          }
          frame "Transmit" {
            n372 = Unbundle By Name(w1049) -> ("Data.Config.DLL_PATH"=w1048:path, "Data.Config.Channel"=w1045:i32, "Data.Config.ChannelMask"=w1044:u16, "Data.Config.ActualPayloadLength"=w1043:u8, "Data.Config.CycleNumber"=w1042:u8, "Data.Config.SlotId"=w1041:u16, "Data.Config.Send_Array"=w1040:u8[])
            n373 = Bundle By Name(cluster=T16 {"FIdxChn"=0, "FChannelMask"=0, "FActualPayloadLength"=0, "FCycleNumber"=0, "FSlotId"=0, "Send_Array"=[1, 2, 3, 4, 5, 6, 7, 8, 9, 10, 11]} ("FR_Transmit"), "FIdxChn"=w1045, "FChannelMask"=w1044, "FActualPayloadLength"=w1043, "FCycleNumber"=w1042, "FSlotId"=w1041, "Send_Array"=w1040) -> (w1046:T16)
            n374 = call "tsapp_transmit_flexray_async.vi"("FR_Transmit"=w1046, "Path"=w1048) -> ("error out"=w1036:errorcluster, "return"=w1037:i32, "Path output"=w1038:path)  [unwired: 6 in]
            n375 = call "error_display.vi"("error in"=w1036, "Action name"=w1034, "return"=w1037, "DLL path"=w1038) -> ("error out"=w1035:errorcluster)  [unwired: 6 in, 1 out]
            n376 = Bundle By Name(cluster=w1049, "error in"=w1035) -> (w1039:T9)
          }
          frame "Connect" {
            n377 = Unbundle By Name(w1060) -> ("Data.AsynCall?"=w1053:bool, "Data.Config.DLL_PATH"=w1059:path, "Data.Config.Channel"=w1058:i32)
            n378 = case shown="假" w1053 {
              tunnel: w1059 -> [w1077 _]
              tunnel: w1058 -> [w1072 _]
              tunnel: [w1069 w1084] -> w1056
              tunnel: [w1064 w1085] -> w1055
              tunnel: string[] ["Connect", "clear_flexray_receive_buffers"] -> [w1063 _]
              tunnel: w1052 -> [_ w1087]
              frame False {
                n379 = call "tsapp_connect.vi"("Path"=w1077) -> ("error out"=w1075:errorcluster, "retuen"=w1068:i32, "Path output"=w1076:path)  [unwired: 8 in]
                n380 = call "tsfifo_enable_receive_fifo.vi"("error in (no error)"=w1075, "Path"=w1076) -> ("error out"=w1074:errorcluster, "Path output"=w1073:path)  [unwired: 8 in]
                n381 = call "tsfifo_clear_flexray_receive_buffers.vi"("error in (no error)"=w1074, "AIdxChn"=w1072, "path in"=w1073) -> ("error out"=w1071:errorcluster, "function return"=w1067:i32, "path out"=w1070:path)  [unwired: 6 in]
                n382 = Build Array(w1068, w1067) -> (w1066:i32[])
                n383 = for {
                  tunnel: w1070 -> [w1082]
                  shift-right: [w1081] -> w1069
                  shift-left: w1071 -> [w1083]
                  tunnel: w1066 -> [w1080] mode=indexing
                  tunnel: [w1079] -> w1065 mode=indexing
                  tunnel: w1063 -> [w1078] mode=indexing
                  n384 = Equal To 0?(x=w1080) -> (x = 0?=w1079:bool)
                  n385 = call "error_display.vi"("error in"=w1083, "Action name"=w1078, "return"=w1080, "DLL path"=w1082) -> ("error out"=w1081:errorcluster)  [unwired: 6 in, 1 out]
                }
                n386 = And Array Elements(Boolean array=w1065) -> (logical AND=w1064:bool)
              }
              frame True {
                n387 = Variant To Data(type=FALSE, Variant=w1087) -> (data=w1085:bool, error out=w1084:errorcluster)  [unwired: 1 in]
              }
            }
            n388 = Bundle By Name(cluster=w1060, "error in"=w1056) -> (w1057:T9)
            n389 = case shown="假" w1055 {
              frame False {
                n390 = local write "Connect ?"(FALSE ("Connect ?")) -> ()
                n391 = disable-structure shown="禁用" {
                  disable-tunnel: "OK" ("按钮名称（“确定”）") -> [w1092 _]
                  disable-tunnel: "Conncet  fail" ("消息") -> [w1091 _]
                  frame Disabled {
                    n392 = One Button Dialog(message=w1091, button name ("OK")=w1092) -> ()  [unwired: 1 out]
                  }
                  frame Enabled {
                  }
                }
              }
              frame True {
                n393 = disable-structure shown="禁用" {
                  disable-tunnel: "OK" ("按钮名称（“确定”）") -> [w1097 _]
                  disable-tunnel: "Conncet  Successful" ("消息") -> [w1096 _]
                  frame Disabled {
                    n394 = One Button Dialog(message=w1096, button name ("OK")=w1097) -> ()  [unwired: 1 out]
                  }
                  frame Enabled {
                  }
                }
                "Connect ?" <- TRUE ("Connect ?")
              }
            }
          }
          frame "Disconnect" {
            n395 = Unbundle By Name(w1105) -> ("Data.AsynCall?"=w1100:bool, "Data.Config.DLL_PATH"=w1104:path)
            n396 = case shown="假" w1100 {
              tunnel: w1104 -> [w1114 _]
              tunnel: [w1113 w1116] -> w1103
              tunnel: [w1109 w1115] -> w1101
              tunnel: w1098 -> [w1108 _]
              tunnel: w1099 -> [_ w1118]
              frame False {
                n397 = call "tsapp_disconnect.vi"("Path"=w1114) -> ("error output"=w1110:errorcluster, "retuen"=w1111:i32, "Path output"=w1112:path)  [unwired: 8 in]
                n398 = call "error_display.vi"("error in"=w1110, "Action name"=w1108, "return"=w1111, "DLL path"=w1112) -> ("error out"=w1109:errorcluster)  [unwired: 6 in, 1 out]
                n399 = Equal To 0?(x=w1111) -> (x = 0?=w1113:bool)
              }
              frame True {
                n400 = Variant To Data(type=FALSE, Variant=w1118) -> (data=w1116:bool, error out=w1115:errorcluster)  [unwired: 1 in]
              }
            }
            n401 = Bundle By Name(cluster=w1105, "error in"=w1101) -> (w1102:T9)
            n402 = case shown="真" w1103 {
              frame False {
              }
              frame True {
                n403 = local write "Connect ?"(FALSE ("Connect ?")) -> ()
              }
            }
          }
          frame "Diagram shown" {
            n404 = control-ref of="本VI"() -> (w1123:refnum<vi>)
            n405 = Variant To Data(type=FALSE, Variant=w1126) -> (data=w1122:bool, error out=w1121:errorcluster)  [unwired: 1 in]
            n406 = property on="Property Node" class="VI"(reference=w1123, error in=w1121, "BDWin.Open"=w1122) -> (error out=w1120:errorcluster)  [unwired: 1 out]
            n407 = Bundle By Name(cluster=w1127, "error in"=w1120) -> (w1124:T9)
          }
          frame "Clear" {
            n408 = Unbundle By Name(w1143) -> ("Data.Config.DLL_PATH"=w1142:path)
            n409 = local read "REC_Channel"() -> (w1141:i32)
            n410 = Bundle By Name(cluster=T15 {"Sender"="", "receiver"="", "message"="", "data"=variant} ("Communication message"), "message"="Clear") -> (w1133:T15)
            n411 = call "tsfifo_clear_flexray_receive_buffers.vi"("AIdxChn"=w1141, "path in"=w1142) -> ("error out"=w1139:errorcluster, "function return"=w1138:i32, "path out"=w1140:path)  [unwired: 7 in]
            n412 = call "error_display.vi"("error in"=w1139, "Action name"=w1137, "return"=w1138, "DLL path"=w1140) -> ("error out"=w1135:errorcluster)  [unwired: 6 in, 1 out]
            n413 = Enqueue Element(queue=w1131, element=w1133, error in (no error)=w1130) -> ()  [unwired: 1 in, 3 out]
            n414 = Bundle By Name(cluster=w1143, "error in"=w1135) -> (w1136:T9)
          }
          frame "DIS_REC" {
            n415 = Variant To Data(type=FALSE, Variant=w1154) -> (data=w1152:bool, error out=w1148:errorcluster)  [unwired: 1 in]
            n416 = Unbundle By Name(w1150) -> ("Data.Config.DLL_PATH"=w1149:path, "Data.Config.REC_Channel"=w1147:i32)
            n417 = case shown="假" w1152 {
              tunnel: w1149 -> [w1158 w1173]
              tunnel: w1148 -> [_ w1172]
              tunnel: w1147 -> [_ w1169]
              tunnel: [w1157 w1160] -> w1146
              frame False {
                n418 = call "tsfifo_enable_receive_fifo.vi"("Path"=w1158) -> ("error out"=w1157:errorcluster)  [unwired: 9 in, 1 out]
                n419 = call "Log.vi"("Data"="EN_REC") -> ()  [unwired: 3 in]
              }
              frame True {
                w1167 = "clear_receive_buffers Successful"  # clear_receive_buffers Successful
                n420 = call "tsfifo_disable_receive_fifo.vi"("error in (no error)"=w1172, "Path"=w1173) -> ("error out"=w1170:errorcluster, "Path output"=w1171:path)  [unwired: 8 in]
                n421 = call "tsfifo_clear_flexray_receive_buffers.vi"("error in (no error)"=w1170, "AIdxChn"=w1169, "path in"=w1171) -> ("error out"=w1160:errorcluster, "function return"=w1161:i32)  [unwired: 6 in, 1 out]
                n422 = Equal To 0?(x=w1161) -> (x = 0?=w1168:bool)
                n423 = Select(t=w1167, s=w1168, f="clear_receive_buffers Fail") -> (s? t:f=w1165:string)
                n424 = Concatenate Strings("DIS_REC" ("string"), "\r", w1165) -> (w1164:string)
                n425 = call "Log.vi"("Data"=w1164) -> ()  [unwired: 3 in]
              }
            }
            n426 = Bundle By Name(cluster=w1150, "error in"=w1146) -> (w1151:T9)
          }
          frame "Creat error" {
            n427 = Variant To Data(type=errorcluster {"status"=FALSE, "code"=0, "source"=""} ("error out"), Variant=w1177) -> (data=w1174:errorcluster)  [unwired: 1 in, 1 out]
            n428 = Bundle By Name(cluster=w1178, "error in"=w1174) -> (w1175:T9)
          }
          frame "Start Log" {
            n429 = Unbundle By Name(w1182) -> ("Data.Config.DLL_PATH"=w1183:path, "Data.Config.BLF_Log_PATH"=w1191:path)
            n430 = Path To String(path=w1191) -> (string=w1190:string)
            n431 = call "tsapp_start_logging.vi"("AFullFileName"=w1190, "路径输入"=w1183) -> ("error out"=w1185:errorcluster, "retuen"=w1184:i32)  [unwired: 7 in, 1 out]
            n432 = Equal To 0?(x=w1184) -> (x = 0?=w1186:bool)
            n433 = Select(t=" Start Log Successful ", s=w1186, f=" Start Log Fail ") -> (s? t:f=w1189:string)
            n434 = Bundle By Name(cluster=w1182, "error in"=w1185) -> (w1181:T9)
            n435 = call "Log.vi"("Data"=w1189) -> ()  [unwired: 3 in]
          }
          frame "Stop Log" {
            n436 = Unbundle By Name(w1195) -> ("Data.Config.DLL_PATH"=w1200:path)
            n437 = call "tsapp_stop_logging.vi"("Path"=w1200) -> ("error out"=w1202:errorcluster, "retuen"=w1201:i32)  [unwired: 8 in, 1 out]
            n438 = Equal To 0?(x=w1201) -> (x = 0?=w1196:bool)
            n439 = Select(t=" Stop Log Successful ", s=w1196, f=" Stop Log Fail ") -> (s? t:f=w1199:string)
            n440 = Bundle By Name(cluster=w1195, "error in"=w1202) -> (w1194:T9)
            n441 = call "Log.vi"("Data"=w1199) -> ()  [unwired: 3 in]
          }
          frame "Import" {
            n442 = Read from Binary File(5:w1209, 7:"Please select a configuration file" ("对话框窗口（打开现有文件）")) -> (0:w1210:errorcluster, 1:w1212:bool, 2:w1211:T9)  [unwired: 4 in, 1 out]
            n443 = case shown="无错误" w1210 {
              selector: w1210 -> [_ w1234]
              tunnel: w1211 -> [w1220 _]
              tunnel: w1212 -> [w1222 _]
              tunnel: w1209 -> [w1221 w1237]
              tunnel: [w1219 w1237] -> w1205
              tunnel: [w1218 w1231] -> w1214
              tunnel: [w1217 _] -> w1206
              frame No Error {
                n444 = case shown="假" w1222 {
                  tunnel: w1221 -> [w1229 w1230]
                  tunnel: w1220 -> [w1228 _]
                  tunnel: [w1226 w1230] -> w1219
                  tunnel: [w1224 _] -> w1218
                  tunnel: ["update" ("按钮名称（“确定”）") _] -> w1217
                  frame False {
                    w1224 = "Import successful" ("消息")
                    n445 = Unbundle By Name(w1228) -> ("Data"=w1227:T18)
                    n446 = Bundle By Name(cluster=w1229, "Data"=w1227) -> (w1226:T9)
                    n447 = One Button Dialog(message=w1224, button name ("OK")="OK" ("按钮名称（“确定”）")) -> ()  [unwired: 1 out]
                  }
                  frame True {
                  }
                }
              }
              frame Error {
                n448 = call <vilib>:"Clear Errors.vi"("error in (no error)"=w1234) -> ()  [unwired: 5 in, 2 out]
                n449 = Unbundle By Name(w1234) -> ("source"=w1235:string)
                n450 = Concatenate Strings("Import Fail" ("消息"), "\r", w1235) -> (w1231:string)
                n451 = One Button Dialog(message=w1231, button name ("OK")="OK" ("按钮名称（“确定”）")) -> ()  [unwired: 1 out]
              }
            }
            n452 = call "Log.vi"("Data"=w1214) -> ()  [unwired: 3 in]
            n453 = Bundle By Name(cluster=T15 {"Sender"="", "receiver"="", "message"="", "data"=variant} ("Communication message"), "message"=w1206) -> (w1207:T15)
          }
          frame "Export" {
            n454 = Write to Binary File(data=w1238, 7:"Please edit the configuration name " ("提示（选择或输入文件路径）")) -> (error out=w1240:errorcluster)  [unwired: 4 in, 2 out]
            n455 = case shown="无错误" w1240 {
              selector: w1240 -> [_ w1247]
              tunnel: [w1244 w1246] -> w1241
              frame No Error {
                w1244 = "Export successful" ("消息")
                n456 = One Button Dialog(message=w1244, button name ("OK")="OK" ("按钮名称（“确定”）")) -> ()  [unwired: 1 out]
              }
              frame Error {
                n457 = Unbundle By Name(w1247) -> ("source"=w1249:string)
                n458 = Concatenate Strings("Export Fail" ("消息"), "\r", w1249) -> (w1246:string)
                n459 = call <vilib>:"Clear Errors.vi"("error in (no error)"=w1247) -> ()  [unwired: 5 in, 2 out]
                n460 = One Button Dialog(message=w1246, button name ("OK")="OK" ("按钮名称（“确定”）")) -> ()  [unwired: 1 out]
              }
            }
            n461 = call "Log.vi"("Data"=w1241) -> ()  [unwired: 3 in]
          }
          frame "update" {
            n462 = Unbundle By Name(w1258) -> ("Data.Config.DLL_PATH"=w1257:path, "Data.Config.Project_PATH"=w1256:path, "Data.Config.BLF_Log_PATH"=w1255:path, "Data.Config.Read message type"=w1254:u16, "Data.Config.Channel"=w1253:i32, "Data.Config.REC_Channel"=w1252:i32)
            n463 = local write "BLF_Log_PATH"(w1255) -> ()
            n464 = local write "Read message type"(w1254) -> ()
            n465 = local write "DLL_PATH"(w1257) -> ()
            n466 = local write "Project_PATH"(w1256) -> ()
            n467 = local write "Channel"(w1253) -> ()
            n468 = local write "REC_Channel"(w1252) -> ()
          }
          frame "Quit" {
            w1264 = T15 {"Sender"="", "receiver"="", "message"="", "data"=variant}  # Message
            w1262 = "Quit" ("y")
            n469 = Bundle By Name(cluster=w1264, "message"=w1262) -> (w1263:T15)
            n470 = Bundle By Name(cluster=T15 {"Sender"="", "receiver"="", "message"="", "data"=variant} ("元素"), "message"=w1262) -> (w1276:T15)
            n471 = call "Log.vi"("Data"=w1262) -> ()  [unwired: 3 in]
            n472 = Generate User Event(user event=w1280, event data cluster=w1263) -> ()  [unwired: 2 in, 2 out]
            n473 = Enqueue Element(queue=w1279, element=w1276, error in (no error)=w1278) -> ()  [unwired: 1 in, 3 out]
            n474 = Unbundle By Name(w1261) -> ("Data.AsynCall?"=w1265:bool, "Data.Config.DLL_PATH"=w1275:path, "Communication message.Sender"=w1267:string)
            n475 = case shown="假" w1265 {
              tunnel: w1275 -> [_ w1289]
              tunnel: [_ w1286] -> w1266
              frame False {
              }
              frame True {
                n476 = call "tsapp_disconnect.vi"("Path"=w1289) -> ("error output"=w1290:errorcluster, "Path output"=w1288:path)  [unwired: 8 in, 1 out]
                n477 = call "finalize_lib_tsmaster.vi"("error in (no error)"=w1290, "Path"=w1288) -> ("error out"=w1287:errorcluster)  [unwired: 8 in, 1 out]
                n478 = call <vilib>:"Clear Errors.vi"("error in (no error)"=w1287) -> ("error out"=w1286:errorcluster)  [unwired: 5 in, 1 out]
              }
            }
            n479 = Current VI's Path() -> (path=w1273:path)
            n480 = Strip Path(path=w1273) -> (stripped path=w1271:path)  [unwired: 1 out]
            n481 = Build Path(base path=w1271, name or relative path="data") -> (appended path=w1270:path)
            n482 = Flush Queue(queue=w1283, error in (no error)=w1281) -> (queue out=w1284:refnum<queue>, error out=w1282:errorcluster)  [unwired: 1 out]
            n483 = call "FlexRay_Configuration_Save.vi"("path"=w1270, "error in (no error)"=w1266, "Config Name"=w1267, "Read/Write"=enum16{"Read", "Write"}."Write", "FlexRay_Data"=w1261) -> ("error in (no error)"=w1268:errorcluster)  [unwired: 4 in, 2 out]
            n484 = Bundle By Name(cluster=w1261, "error in"=w1268) -> (w1274:T9)
          }
        }
        n485 = Unbundle By Name(w270) -> ("error in"=w269:errorcluster)
        n486 = Unbundle By Name(w274) -> ("message"=w273:string)
        n487 = call "error_collect.vi"("error in (no error)"=w269) -> ("error IO"=w267:errorcluster)  [unwired: 10 in]
        n488 = case shown="\"default\", 默认" w273 {
          tunnel: w280 -> [w290 w292]
          tunnel: w279 -> [w289 w291]
          tunnel: w274 -> [w288 _]
          tunnel: [w287 w292] -> w277
          tunnel: [w286 w291] -> w276
          frame "default", Default {
            n489 = Enqueue Element(queue=w290, element=w288, error in (no error)=w289) -> (queue out=w287:refnum<queue>, error out=w286:errorcluster)  [unwired: 1 in, 1 out]
          }
          frame "" {
          }
        }
        n490 = Bundle By Name(cluster=w270, "error in"=w267) -> (w268:T9)
      }
      n491 = while {
        tunnel: w86 -> [w1300]
        tunnel: w82 -> [w1298]
        tunnel: w66 -> [w1294]
        tunnel: w80 -> [w1293]
        tunnel: [w1292] -> w79
        tunnel: w78 -> [w1291]
        tunnel: [w1291] -> w77
        stop <- w1301 stop-if-true
        # "Event Handling Loop"
        n492 = event shown="[28] \"Signals\": 值改变" {
          selector: w1293 -> [_ _ _ _ _ _ _ _ _ _ _ _ _ _ _ _ _ _ _ _ _ _ _ _ _ _ _ _ _ _ _ _ _ _]
          dyn-events: [_ _ _ _ _ _ _ _ _ _ _ _ _ _ _ _ _ _ _ _ _ _ _ _ _ _ _ _ _ _ _ _ _ _] -> w1292
          timeout: _ -> [_ _ _ _ _ _ _ _ _ _ _ _ _ _ _ _ _ _ _ _ _ _ _ _ _ _ _ _ _ _ _ _ _ _]
          tunnel: [_ _ _ _ _ _ _ _ _ _ _ _ _ _ _ _ _ _ _ _ _ _ _ _ _ w1467 w1483 _ _ _ _ _ _ _] -> w1301
          tunnel: w1300 -> [w1311 w1318 w1325 w1332 w1339 w1346 w1351 w1358 w1363 w1370 w1377 w1384 w1391 w1398 w1405 w1412 w1419 w1424 w1429 w1434 w1439 w1444 w1451 w1458 w1463 w1469 w1486 w1493 w1500 w1507 w1512 w1517 w1522 w1527]
          tunnel: [w1311 w1318 w1325 w1332 w1339 w1346 w1351 w1358 w1363 w1370 w1377 w1384 w1391 w1398 w1405 w1412 w1419 w1424 w1429 w1434 w1439 w1444 w1451 w1458 w1463 w1469 w1484 w1493 w1500 w1507 w1512 w1517 w1522 w1527] -> w1299
          tunnel: [T15 {"Sender"="", "receiver"="", "message"="", "data"=variant} ("Communication message") w1314 w1320 w1327 w1334 w1341 w1347 w1353 w1359 w1365 w1372 w1379 w1386 w1393 w1400 w1407 w1414 w1420 w1425 w1430 w1435 w1440 w1447 w1453 w1461 _ _ w1488 w1495 w1503 w1508 w1513 w1518 w1523] -> w1296
          tunnel: [w1310 w1317 w1324 w1331 w1338 w1345 w1350 w1357 w1362 w1369 w1376 w1383 w1390 w1397 w1404 w1411 w1418 w1423 w1428 w1433 w1438 w1443 w1450 w1457 w1459 w1466 w1482 w1492 w1499 w1506 w1511 w1516 w1521 w1526] -> w1297
          tunnel: w1298 -> [w1310 w1317 w1324 w1331 w1338 w1345 w1350 w1357 w1362 w1369 w1376 w1383 w1390 w1397 w1404 w1411 w1418 w1423 w1428 w1433 w1438 w1443 w1450 w1457 w1459 w1466 w1482 w1492 w1499 w1506 w1511 w1516 w1521 w1526]
          tunnel: w1294 -> [_ _ _ _ _ _ _ _ _ _ _ _ _ _ _ _ _ _ _ _ _ _ _ _ _ _ _ _ _ _ _ _ _ _]
          event Timeout {
            n493 = event-data() -> ()  [unwired: 1 in, 3 out]
          }
          event "DLL_PATH": Value Change {
            n494 = event-data() -> ("NewVal"=w1312:path)  [unwired: 1 in, 5 out]
            n495 = To Variant(anything=w1312) -> (Variant=w1313:variant)
            n496 = Bundle By Name(cluster=T15 {"Sender"="", "receiver"="", "message"="", "data"=variant} ("Communication message"), "message"="DLL_PATH" ("Sender"), "data"=w1313) -> (w1314:T15)
          }
          event "Project_PATH": Value Change {
            n497 = event-data() -> ("NewVal"=w1319:path)  [unwired: 1 in, 5 out]
            n498 = To Variant(anything=w1319) -> (Variant=w1321:variant)
            n499 = Bundle By Name(cluster=T15 {"Sender"="", "receiver"="", "message"="", "data"=variant} ("Communication message"), "message"="Project_PATH" ("Sender"), "data"=w1321) -> (w1320:T15)
          }
          event "BLF_Log_PATH": Value Change {
            n500 = event-data() -> ("NewVal"=w1326:path)  [unwired: 1 in, 5 out]
            n501 = To Variant(anything=w1326) -> (Variant=w1328:variant)
            n502 = Bundle By Name(cluster=T15 {"Sender"="", "receiver"="", "message"="", "data"=variant} ("Communication message"), "message"="BLF_Log_PATH" ("Sender"), "data"=w1328) -> (w1327:T15)
          }
          event "XML Path": Value Change {
            n503 = event-data() -> ("NewVal"=w1333:path)  [unwired: 1 in, 5 out]
            n504 = To Variant(anything=w1333) -> (Variant=w1335:variant)
            n505 = Bundle By Name(cluster=T15 {"Sender"="", "receiver"="", "message"="", "data"=variant} ("Communication message"), "message"="XML Path" ("Sender"), "data"=w1335) -> (w1334:T15)
          }
          event "XML loading channel": Value Change {
            n506 = event-data() -> ("NewVal"=w1340:i32)  [unwired: 1 in, 5 out]
            n507 = To Variant(anything=w1340) -> (Variant=w1342:variant)
            n508 = Bundle By Name(cluster=T15 {"Sender"="", "receiver"="", "message"="", "data"=variant} ("Communication message"), "message"="XML loading channel" ("Sender"), "data"=w1342) -> (w1341:T15)
          }
          event "Load_XML": Value Change {
            n509 = event-data() -> ()  [unwired: 1 in, 6 out]
            n510 = Bundle By Name(cluster=T15 {"Sender"="", "receiver"="", "message"="", "data"=variant} ("Communication message"), "message"="Load_XML" ("Sender")) -> (w1347:T15)
          }
          event "Tree control": Mouse Up {
            n511 = event-data() -> ("CtlRef"=w1352:refnum<vi>)  [unwired: 1 in, 7 out]
            n512 = To Variant(anything=w1352) -> (Variant=w1354:variant)
            n513 = Bundle By Name(cluster=T15 {"Sender"="", "receiver"="", "message"="", "data"=variant} ("Communication message"), "message"="XML_Define", "data"=w1354) -> (w1353:T15)
          }
          event "Unload": Value Change {
            n514 = event-data() -> ()  [unwired: 1 in, 6 out]
            n515 = Bundle By Name(cluster=T15 {"Sender"="", "receiver"="", "message"="", "data"=variant} ("Communication message"), "message"="Unload" ("Sender")) -> (w1359:T15)
          }
          event "Read message type": Value Change {
            n516 = event-data() -> ("NewVal"=w1364:u16)  [unwired: 1 in, 5 out]
            n517 = To Variant(anything=w1364) -> (Variant=w1366:variant)
            n518 = Bundle By Name(cluster=T15 {"Sender"="", "receiver"="", "message"="", "data"=variant} ("Communication message"), "message"="Read message type" ("Sender"), "data"=w1366) -> (w1365:T15)
          }
          event "Channel": Value Change {
            n519 = event-data() -> ("NewVal"=w1371:i32)  [unwired: 1 in, 5 out]
            n520 = To Variant(anything=w1371) -> (Variant=w1373:variant)
            n521 = Bundle By Name(cluster=T15 {"Sender"="", "receiver"="", "message"="", "data"=variant} ("Communication message"), "message"="Channel" ("Sender"), "data"=w1373) -> (w1372:T15)
          }
          event "REC_Channel": Value Change {
            n522 = event-data() -> ("NewVal"=w1378:i32)  [unwired: 1 in, 5 out]
            n523 = To Variant(anything=w1378) -> (Variant=w1380:variant)
            n524 = Bundle By Name(cluster=T15 {"Sender"="", "receiver"="", "message"="", "data"=variant} ("Communication message"), "message"="REC_Channel" ("Sender"), "data"=w1380) -> (w1379:T15)
          }
          event "CycleNumber": Value Change {
            n525 = event-data() -> ("NewVal"=w1385:u8)  [unwired: 1 in, 5 out]
            n526 = To Variant(anything=w1385) -> (Variant=w1387:variant)
            n527 = Bundle By Name(cluster=T15 {"Sender"="", "receiver"="", "message"="", "data"=variant} ("Communication message"), "message"="CycleNumber" ("Sender"), "data"=w1387) -> (w1386:T15)
          }
          event "ActualPayloadLength": Value Change {
            n528 = event-data() -> ("NewVal"=w1392:u8)  [unwired: 1 in, 5 out]
            n529 = To Variant(anything=w1392) -> (Variant=w1394:variant)
            n530 = Bundle By Name(cluster=T15 {"Sender"="", "receiver"="", "message"="", "data"=variant} ("Communication message"), "message"="ActualPayloadLength" ("Sender"), "data"=w1394) -> (w1393:T15)
          }
          event "SlotId": Value Change {
            n531 = event-data() -> ("NewVal"=w1399:u16)  [unwired: 1 in, 1 out]
            n532 = To Variant(anything=w1399) -> (Variant=w1401:variant)
            n533 = Bundle By Name(cluster=T15 {"Sender"="", "receiver"="", "message"="", "data"=variant} ("Communication message"), "message"="SlotId" ("Sender"), "data"=w1401) -> (w1400:T15)
          }
          event "ChannelMask": Value Change {
            n534 = event-data() -> ("NewVal"=w1406:u16)  [unwired: 1 in, 5 out]
            n535 = To Variant(anything=w1406) -> (Variant=w1408:variant)
            n536 = Bundle By Name(cluster=T15 {"Sender"="", "receiver"="", "message"="", "data"=variant} ("Communication message"), "message"="ChannelMask" ("Sender"), "data"=w1408) -> (w1407:T15)
          }
          event "Send_Array": Value Change {
            n537 = event-data() -> ("NewVal"=w1413:u8[])  [unwired: 1 in, 5 out]
            n538 = To Variant(anything=w1413) -> (Variant=w1415:variant)
            n539 = Bundle By Name(cluster=T15 {"Sender"="", "receiver"="", "message"="", "data"=variant} ("Communication message"), "message"="Send_Array" ("Sender"), "data"=w1415) -> (w1414:T15)
          }
          event "Transmit": Value Change {
            n540 = event-data() -> ()  [unwired: 1 in, 6 out]
            n541 = Bundle By Name(cluster=T15 {"Sender"="", "receiver"="", "message"="", "data"=variant} ("Communication message"), "message"="Transmit" ("Sender")) -> (w1420:T15)
          }
          event "Config": Value Change {
            n542 = event-data() -> ()  [unwired: 1 in, 6 out]
            n543 = Bundle By Name(cluster=T15 {"Sender"="", "receiver"="", "message"="", "data"=variant} ("Communication message"), "message"="Init" ("Sender")) -> (w1425:T15)
          }
          event "Connect": Value Change {
            n544 = event-data() -> ()  [unwired: 1 in, 6 out]
            n545 = Bundle By Name(cluster=T15 {"Sender"="", "receiver"="", "message"="", "data"=variant} ("Communication message"), "message"="Connect" ("Sender")) -> (w1430:T15)
          }
          event "Disconnect": Value Change {
            n546 = event-data() -> ()  [unwired: 1 in, 6 out]
            n547 = Bundle By Name(cluster=T15 {"Sender"="", "receiver"="", "message"="", "data"=variant} ("Communication message"), "message"="Disconnect" ("Sender")) -> (w1435:T15)
          }
          event "Clear": Value Change {
            n548 = event-data() -> ()  [unwired: 1 in, 6 out]
            n549 = Bundle By Name(cluster=T15 {"Sender"="", "receiver"="", "message"="", "data"=variant} ("Communication message"), "message"="Clear" ("Sender")) -> (w1440:T15)
          }
          event "DIS_REC": Value Change {
            n550 = event-data() -> ("NewVal"=w1446:bool)  [unwired: 1 in, 5 out]
            n551 = To Variant(anything=w1446) -> (Variant=w1445:variant)
            n552 = Bundle By Name(cluster=T15 {"Sender"="", "receiver"="", "message"="", "data"=variant} ("Communication message"), "message"="DIS_REC" ("Sender"), "data"=w1445) -> (w1447:T15)
          }
          event "Diagram shown": Value Change {
            n553 = event-data() -> ("NewVal"=w1452:bool)  [unwired: 1 in, 5 out]
            n554 = To Variant(anything=w1452) -> (Variant=w1454:variant)
            n555 = Bundle By Name(cluster=T15 {"Sender"="", "receiver"="", "message"="", "data"=variant} ("Communication message"), "message"="Diagram shown" ("Sender"), "data"=w1454) -> (w1453:T15)
          }
          event "Quit": Value Change {
            n556 = event-data() -> ()  [unwired: 1 in, 6 out]
            n557 = Bundle By Name(cluster=T15 {"Sender"="", "receiver"="", "message"="", "data"=variant} ("Communication message"), "message"="Quit" ("Sender")) -> (w1461:T15)
          }
          event User Event {
            n558 = event-data() -> ("message"=w1465:string, "data"=w1464:variant)  [unwired: 1 in, 2 out]
            n559 = case shown="\"Messages\"" w1465 {
              tunnel: w1464 -> [_ w1478 w1481]
              frame Default {
              }
              frame "Messages" {
                n560 = Variant To Data(type=T17 {"Frame_Properties"={"FDBIndex"=0, "FECUIndex"=0, "FFrameIndex"=0, "FIsTx"=0, "FReserved1"=0, "FCycleTimeMs"=0, "TSignalType"=0, "FCANIsDataFrame"=0, "FCANIsStdFrame"=0, "FCANIsEdl"=0, "FCANIsBrs"=0, "FCANIdentifier"=0, "FCANDLC"=0, "FCANDataBytes"=0, "FLINIdentifier"=0, "FLINDLC"=0, "FFRChannelMask"=0, "FFRBaseCycle"=0, "FFRCycleRepetition"=0, "FFRIsStartupFrame"=0, "FFRSlotId"=0, "FFRDLC"=0, "FFRCycleMask"=0, "FSignalCount"=0, "FName"={"数值"=0, "数值 2"=0, "数值 3"=0, "数值 4"=0, "数值 5"=0, "数值 6"=0, "数值 7"=0, "数值 8"=0, "数值 9"=0, "数值 10"=0, "数值 11"=0, "数值 12"=0, "数值 13"=0, "数值 14"=0, "数值 15"=0, "数值 16"=0, "数值 17"=0, "数值 18"=0, "数值 19"=0, "数值 20"=0, "数值 21"=0, "数值 22"=0, "数值 23"=0, "数值 24"=0, "数值 25"=0, "数值 26"=0, "数值 27"=0, "数值 28"=0, "数值 29"=0, "数值 30"=0, "数值 31"=0, "数值 32"=0, "数值 33"=0, "数值 34"=0, "数值 35"=0, "数值 36"=0, "数值 37"=0, "数值 38"=0, "数值 39"=0, "数值 40"=0, "数值 41"=0, "数值 42"=0, "数值 43"=0, "数值 44"=0, "数值 45"=0, "数值 46"=0, "数值 47"=0, "数值 48"=0, "数值 49"=0, "数值 50"=0, "数值 51"=0, "数值 52"=0, "数值 53"=0, "数值 54"=0, "数值 55"=0, "数值 56"=0, "数值 57"=0, "数值 58"=0, "数值 59"=0, "数值 60"=0, "数值 61"=0, "数值 62"=0, "数值 63"=0, "数值 64"=0}, "FComment"={"数值"=0, "数值 2"=0, "数值 3"=0, "数值 4"=0, "数值 5"=0, "数值 6"=0, "数值 7"=0, "数值 8"=0, "数值 9"=0, "数值 10"=0, "数值 11"=0, "数值 12"=0, "数值 13"=0, "数值 14"=0, "数值 15"=0, "数值 16"=0, "数值 17"=0, "数值 18"=0, "数值 19"=0, "数值 20"=0, "数值 21"=0, "数值 22"=0, "数值 23"=0, "数值 24"=0, "数值 25"=0, "数值 26"=0, "数值 27"=0, "数值 28"=0, "数值 29"=0, "数值 30"=0, "数值 31"=0, "数值 32"=0, "数值 33"=0, "数值 34"=0, "数值 35"=0, "数值 36"=0, "数值 37"=0, "数值 38"=0, "数值 39"=0, "数值 40"=0, "数值 41"=0, "数值 42"=0, "数值 43"=0, "数值 44"=0, "数值 45"=0, "数值 46"=0, "数值 47"=0, "数值 48"=0, "数值 49"=0, "数值 50"=0, "数值 51"=0, "数值 52"=0, "数值 53"=0, "数值 54"=0, "数值 55"=0, "数值 56"=0, "数值 57"=0, "数值 58"=0, "数值 59"=0, "数值 60"=0, "数值 61"=0, "数值 62"=0, "数值 63"=0, "数值 64"=0}}, "signal_array"=[]} ("Frame"), Variant=w1478) -> (data=w1476:T17)  [unwired: 1 in, 1 out]
                n561 = Unbundle By Name(w1476) -> ("Frame_Properties.FFRSlotId"=w1475:u16, "Frame_Properties.FFRDLC"=w1474:u16, "Frame_Properties.FFRChannelMask"=w1473:u8, "Frame_Properties.FFRBaseCycle"=w1472:u8, "Frame_Properties.FFRCycleRepetition"=w1471:u8)
                n562 = Add(x=w1472, y=w1471) -> (x+y=w1470:u8)
                n563 = property on="SlotId" class="DigNum (严格)"("Val(Sgnl)"=w1475) -> ()  [unwired: 2 in, 2 out]
                n564 = property on="ActualPayloadLength" class="DigNum (严格)"("Val(Sgnl)"=w1474) -> ()  [unwired: 2 in, 2 out]
                n565 = property on="ChannelMask" class="Ring (严格)"("Val(Sgnl)"=w1473) -> ()  [unwired: 2 in, 2 out]
                n566 = property on="CycleNumber" class="DigNum (严格)"("Val(Sgnl)"=w1470) -> ()  [unwired: 2 in, 2 out]
              }
              frame "Signals" {
                n567 = Variant To Data(type=u8[] [], Variant=w1481) -> (data=w1479:u8[])  [unwired: 1 in, 1 out]
                n568 = property on="Send_Array" class="Arr (严格)"("Val(Sgnl)"=w1479) -> ()  [unwired: 2 in, 2 out]
              }
            }
            n569 = Equal?(x=w1465, y="Quit") -> (x = y?=w1467:bool)
          }
          event Panel Close? {
            w1483 = TRUE ("放弃？")
            n570 = event-data() -> ()  [unwired: 1 in, 1 out]
            n571 = Enqueue Element(queue=w1486, element=T15 {"Sender"="", "receiver"="", "message"="Quit", "data"=variant} ("Communication message")) -> (queue out=w1484:refnum<queue>)  [unwired: 2 in, 2 out]
            n572 = event-data("Discard?"=w1483) -> ()  [unwired: 1 in, 1 out]
          }
          event "Messages": Value Change {
            n573 = event-data() -> ("NewVal"=w1487:string)  [unwired: 1 in, 3 out]
            n574 = To Variant(anything=w1487) -> (Variant=w1489:variant)
            n575 = Bundle By Name(cluster=T15 {"Sender"="", "receiver"="", "message"="", "data"=variant} ("Communication message"), "message"="Messages" ("Sender"), "data"=w1489) -> (w1488:T15)
          }
          event "Signals": Value Change {
            n576 = event-data() -> ("NewVal"=w1494:string[][])  [unwired: 1 in, 3 out]
            n577 = To Variant(anything=w1494) -> (Variant=w1496:variant)
            n578 = Bundle By Name(cluster=T15 {"Sender"="", "receiver"="", "message"="", "data"=variant} ("Communication message"), "message"="Signals" ("Sender"), "data"=w1496) -> (w1495:T15)
          }
          event "Creat error": Value Change {
            n579 = event-data() -> ()  [unwired: 1 in, 6 out]
            n580 = To Variant(anything=errorcluster {"status"=TRUE, "code"=709394, "source"="This is a error demo"}) -> (Variant=w1501:variant)
            n581 = Bundle By Name(cluster=T15 {"Sender"="", "receiver"="", "message"="", "data"=variant} ("Communication message"), "message"="Creat error" ("Sender"), "data"=w1501) -> (w1503:T15)
          }
          event "Start Log": Value Change {
            n582 = event-data() -> ()  [unwired: 1 in, 6 out]
            n583 = Bundle By Name(cluster=T15 {"Sender"="", "receiver"="", "message"="", "data"=variant} ("Communication message"), "message"="Start Log" ("Sender")) -> (w1508:T15)
          }
          event "Stop Log": Value Change {
            n584 = event-data() -> ()  [unwired: 1 in, 6 out]
            n585 = Bundle By Name(cluster=T15 {"Sender"="", "receiver"="", "message"="", "data"=variant} ("Communication message"), "message"="Stop Log" ("Sender")) -> (w1513:T15)
          }
          event "Import": Value Change {
            n586 = event-data() -> ()  [unwired: 1 in, 6 out]
            n587 = Bundle By Name(cluster=T15 {"Sender"="", "receiver"="", "message"="", "data"=variant} ("Communication message"), "message"="Import" ("Sender")) -> (w1518:T15)
          }
          event "Export": Value Change {
            n588 = event-data() -> ()  [unwired: 1 in, 6 out]
            n589 = Bundle By Name(cluster=T15 {"Sender"="", "receiver"="", "message"="", "data"=variant} ("Communication message"), "message"="Export" ("Sender")) -> (w1523:T15)
          }
        }
        n590 = Unbundle By Name(w1296) -> ("message"=w1295:string)
        n591 = case shown="\"default\", 默认" w1295 {
          tunnel: w1299 -> [w1306 w1308]
          tunnel: w1297 -> [w1305 w1307]
          tunnel: w1296 -> [w1304 _]
          tunnel: [w1303 w1308] -> _
          tunnel: [w1302 w1307] -> _
          frame "default", Default {
            n592 = Enqueue Element(queue=w1306, element=w1304, error in (no error)=w1305) -> (queue out=w1303:refnum<queue>, error out=w1302:errorcluster)  [unwired: 1 in, 1 out]
          }
          frame "" {
          }
        }
      }
    }
  }
  n593 = Release Queue(queue=w6, error in (no error)=w5) -> ()  [unwired: 1 in, 3 out]
  n594 = Release Queue(queue=w15, error in (no error)=w14) -> (error out=w13:errorcluster)  [unwired: 1 in, 2 out]
  n595 = Destroy User Event(user event=w8) -> (error out=w9:errorcluster)  [unwired: 1 in]
  n596 = property class="App"(error in=w13) -> (error out=w12:errorcluster, "App.Kind"=w11:T19)  [unwired: 1 in, 1 out]
  n597 = Unregister For Events(event registration refnum=w10, error in=w9) -> ()  [unwired: 1 out]
  n598 = Bundle By Name(cluster=w7, "Communication message"=w1) -> (→"FlexRay_Data":T9)
  n599 = case shown="\"Run Time System\"" w11 {
    tunnel: w12 -> [_ _ w1528 _ _ _ _]
    frame "invalid app kind", Default {
    }
    frame "Development System" {
    }
    frame "Run Time System" {
      n600 = invoke class="VI" method="FP.Close"(error in=w1528) -> ()  [unwired: 2 in, 3 out]
    }
    frame "Student Edition" {
    }
    frame "Embedded LabVIEW" {
    }
    frame "Evaluation" {
    }
    frame "Custom" {
    }
  }
